vi "COD主界面（列队使用）.vi"() -> (8 "多列列表框":i32(listbox))   [LabVIEW 2016, in "斯坦道CODMn.lvlib"]
uses:
  <vilib>/Analysis/6fits.llb/Curve Fitting Criteria.ctl
  <vilib>/Utility/miscctls.llb/LVPointTypeDef.ctl
  <vilib>/Utility/config.llb/Read Key (I32).vi
  <vilib>/Utility/config.llb/Read Key (Double).vi
  <vilib>/Utility/config.llb/Read Key (Boolean).vi
  <vilib>/Utility/config.llb/Write Key (Double).vi
  <vilib>/Utility/config.llb/Write Key (Boolean).vi
  <vilib>/Utility/config.llb/Write Key (I32).vi
  <vilib>/Waveform/WDTFileIO.llb/Read Waveform from File.vi
  <vilib>/ptbypt/NI_PtbyPt.lvlib
  <vilib>/Utility/config.llb/NI_LVConfig.lvlib
  <vilib>/Analysis/NI_AALPro.lvlib
panel:
  in  "远程校准量程":enum16{"L", "H"}(ring)
  in  "远程自动校准浓度":dbl
  in  "仪器参数":bool
  out "CODMn序列号":string
  out "CODMn软件版本：":string
  in  "标样核查量程选择":enum32{"H", "L", "AUTO"}(ring)=enum."AUTO"
  in  "标样浓度":dbl
  in  "零点核查量程选择":enum32{"H", "L", "AUTO"}(ring)=enum."AUTO"
  in  "零点核查浓度":dbl
  out "序列号":string
  in  "采水泵排液时间/s:":i32
  in  "采水泵润洗时间/s:":i32
  in  "采水泵沉淀时间/s:":i32
  in  "采水泵进样时间/s:":i32
  in  "常规版/认证版":enum16{"常规版", "认证版", "浮台版"}(ring)
  in  "释放串口":bool
  in  "打开串口":bool
  in  "保存参数":dbl[](array[numeric])
  out "报警数字":i16
  out "CODMn工作状态":T1(ring)
  out "ORP-K":string
  out "ORP-B":string
  out "ORP-A":string
  out "x = y?":bool
  out "稀释倍数解释":string
  in  "跨度量程选择":enum32{"H", "L", "AUTO"}(ring)=enum."AUTO"
  in  "跨度液浓度":dbl
  in  "水样":dbl
  in  "蒸馏水":dbl
  in  "标液":dbl
  in  "质控样":dbl
  in  "加标回收":dbl
  in  "草酸钠":dbl
  in  "高锰酸钾":dbl
  in  "硫酸":dbl
  out "量程解释说明":string
  in  "高切低阈值:":dbl
  in  "低切高阈值:":dbl
  in  "自动切换量程:":enum16{"关闭", "自动切换测一次", "自动切换测两次"}(ring)
  in  "修正系数":dbl
  in  "标准液浓度":dbl
  in  "温度":dbl
  in  "恒温时间":dbl
  in  "基本量程":enum16{"L", "H"}(ring)
  in  "CODMn零点核查选择":enum16{"零点核查走纯水管", "零点核查走零漂管"}(ring)
  in  "锁定按钮":bool
  in  "低量程稀释倍数:":i8=1
  in  "高量程稀释倍数:":i8=2
  in  "一键写入":bool
  in  "测量模式(公式)":u16(ring)=1 items=["水样测试"=1, "标样核查"=2, "零点核查"=3, "跨度核查"=4, "空白测试"=5, "平行样"=6, "加标回收"=7]
  out "基本量程(显示)":string
  out "测量模式(显示)":string
  out "数据时间":string
  out "断电排液标记":bool
  out "COM":string
  in  "启用5":bool
  in  "校准5":bool
  in  "泵滴定数5":dbl
  in  "浓度5":dbl
  in  "启用4":bool
  in  "校准4":bool
  in  "泵滴定数4":dbl
  in  "浓度4":dbl
  out "波形时间":timestamp
  in  "历史波形":bool
  out "滴定数-ORP值":u16[](array[numeric]) caption="数组"
  in  "关闭 3":bool
  in  "滴定曲线":bool
  out "ORP滴定曲线":u16[](graph)
  out "空白测试标记":bool
  out "跨度核查标记":bool
  out "启动选择 2":u16(ring) items=["水样测试", "标样核查", "零点核查", "跨度核查", "空白测试", "加标回收", "平行样", "校零", "校标"]
  in  "量程选择":enum16{"低量程", "高量程", "0-2量程"}(ring)
  in  "手动控制":bool
  in  "选用水样":enum16{"葡萄糖", "草酸钠"}(ring)
  in  "方程系数":cluster{"K":dbl, "b":dbl, "X^2":dbl} {"X^2" format="%#.6g"; "b" format="%#.6g"; "K" format="%#.6g"}
  out "多项式系数":dbl[](array[numeric])
  out "XY图":cluster{"X Values":dbl[], "Y Values":dbl[]}[](graph)
  in  "模型":enum32{"线性", "多项式"}(ring)
  out "启动时间":timestamp format="%<%Y/%m/%d %H:%M:%S>T"
  in  "关闭 2":bool
  out "r^2":dbl format="%.8g"
  out "拟合公式":string
  out "b":dbl format="%#.4g"
  out "K":dbl format="%#.4f"
  out "当前校准":i32
  in  "启用3":bool
  in  "启用2":bool
  in  "启用1":bool
  in  "校准3":bool
  in  "校准2":bool
  in  "校准1":bool
  in  "泵滴定数3":dbl
  in  "泵滴定数2":dbl
  in  "泵滴定数1":dbl
  in  "浓度3":dbl
  in  "浓度2":dbl
  in  "浓度1":dbl
  in  "写入":bool
  out "零点核查标记":bool
  out "排液故障":bool
  out "进水样超量程":bool
  out "标样核查标记":bool
  out "平行样测量":bool
  out "加标回收测量":bool
  out "质控样测量":bool
  out "待机":bool
  out "校标错误":bool
  out "校零错误":bool
  out "测量错误":bool
  out "草酸钠报警":bool
  out "高锰酸钾报警":bool
  out "加热故障":bool
  out "温控器故障":bool
  out "ORP故障":bool
  out "排液标记":bool
  out "故障标记":bool
  out "校标标记":bool
  out "校零标记":bool
  out "通讯状态":bool
  out "水样测量":bool
  in  "读取":bool
  in  "返回":bool
  in  "校准配置":bool
  in  "零点泵计量数 2":dbl
  in  "标度泵计量数 2":dbl
  out "标度滴定值":dbl
  out "零点滴定值":dbl
  in  "保存":bool
  in  "关闭":bool
  out "仪器时间":timestamp format="%<%Y/%m/%d %H:%M:%S>T"
  out "秒":u16
  out "分":u16
  out "COD浓度（mg/L)":dbl format="%.2g"
  out "进样管":dbl
  out "高锰酸钾":dbl
  out "草酸钠":dbl
  out "硫酸":dbl
  out "ORP显示":dbl
  out "温度":dbl
  out "加热":bool
  out "搅拌":bool
  out "进硫酸":bool
  out "进加标回收样":bool
  out "进零点核查样":bool
  out "进标液":bool
  out "进蒸馏水":bool
  out "进水样":bool
  out "进草酸钠":bool
  out "进高锰酸钾":bool
  out "定时启动":bool
  in  "启动":bool
  in  "故障清除":bool
  in  "参数配置":bool
  in  "停止":bool
  in  "单步启动":bool
  out "系统时间":timestamp
  in  "时间校准":bool
  out "模式（受控）":u16
  # "测量时间："
  # "(水样~加标回收)"
  # "mV"
  # "℃"
  # "注：遇到加热故障和排液故障时仪器不能正常启动，\n必须排查故障并点击报警清除按钮方可运行。"
  # "mg/L"
  # "基本参数设置"
  # "校零校标结果"
  # "泵计量参数设置"
  # "校零结果："
  # "校零滴定值："
  # "加热恒温温度(℃):"
  # "水样："
  # "高锰酸钾："
  # "校标结果："
  # "标度滴定值："
  # "恒温时间(分钟):"
  # "草酸钠："
  # "蒸馏水："
  # "零点泵计量值："
  # "标准液浓度(mg/L):"
  # "硫酸："
  # "标液："
  # "标度泵计量值："
  # "修正系数："
  # "跨度核查浓度："
  # "零点核查样:"
  # "基本量程(L、H)可选:"
  # "跨度量程选择："
  # "加标回收样："
  # "零点核查浓度："
  # "标样浓度："
  # "零点量程选择："
  # "标样量程选择："
  # "远程校准配置区"
  # "公式读取写入区"
  # "mg/L"
  # "是否启用"
  # "泵滴定数"
  # "浓度"
  # "辅\n助\n计\n算\n区"
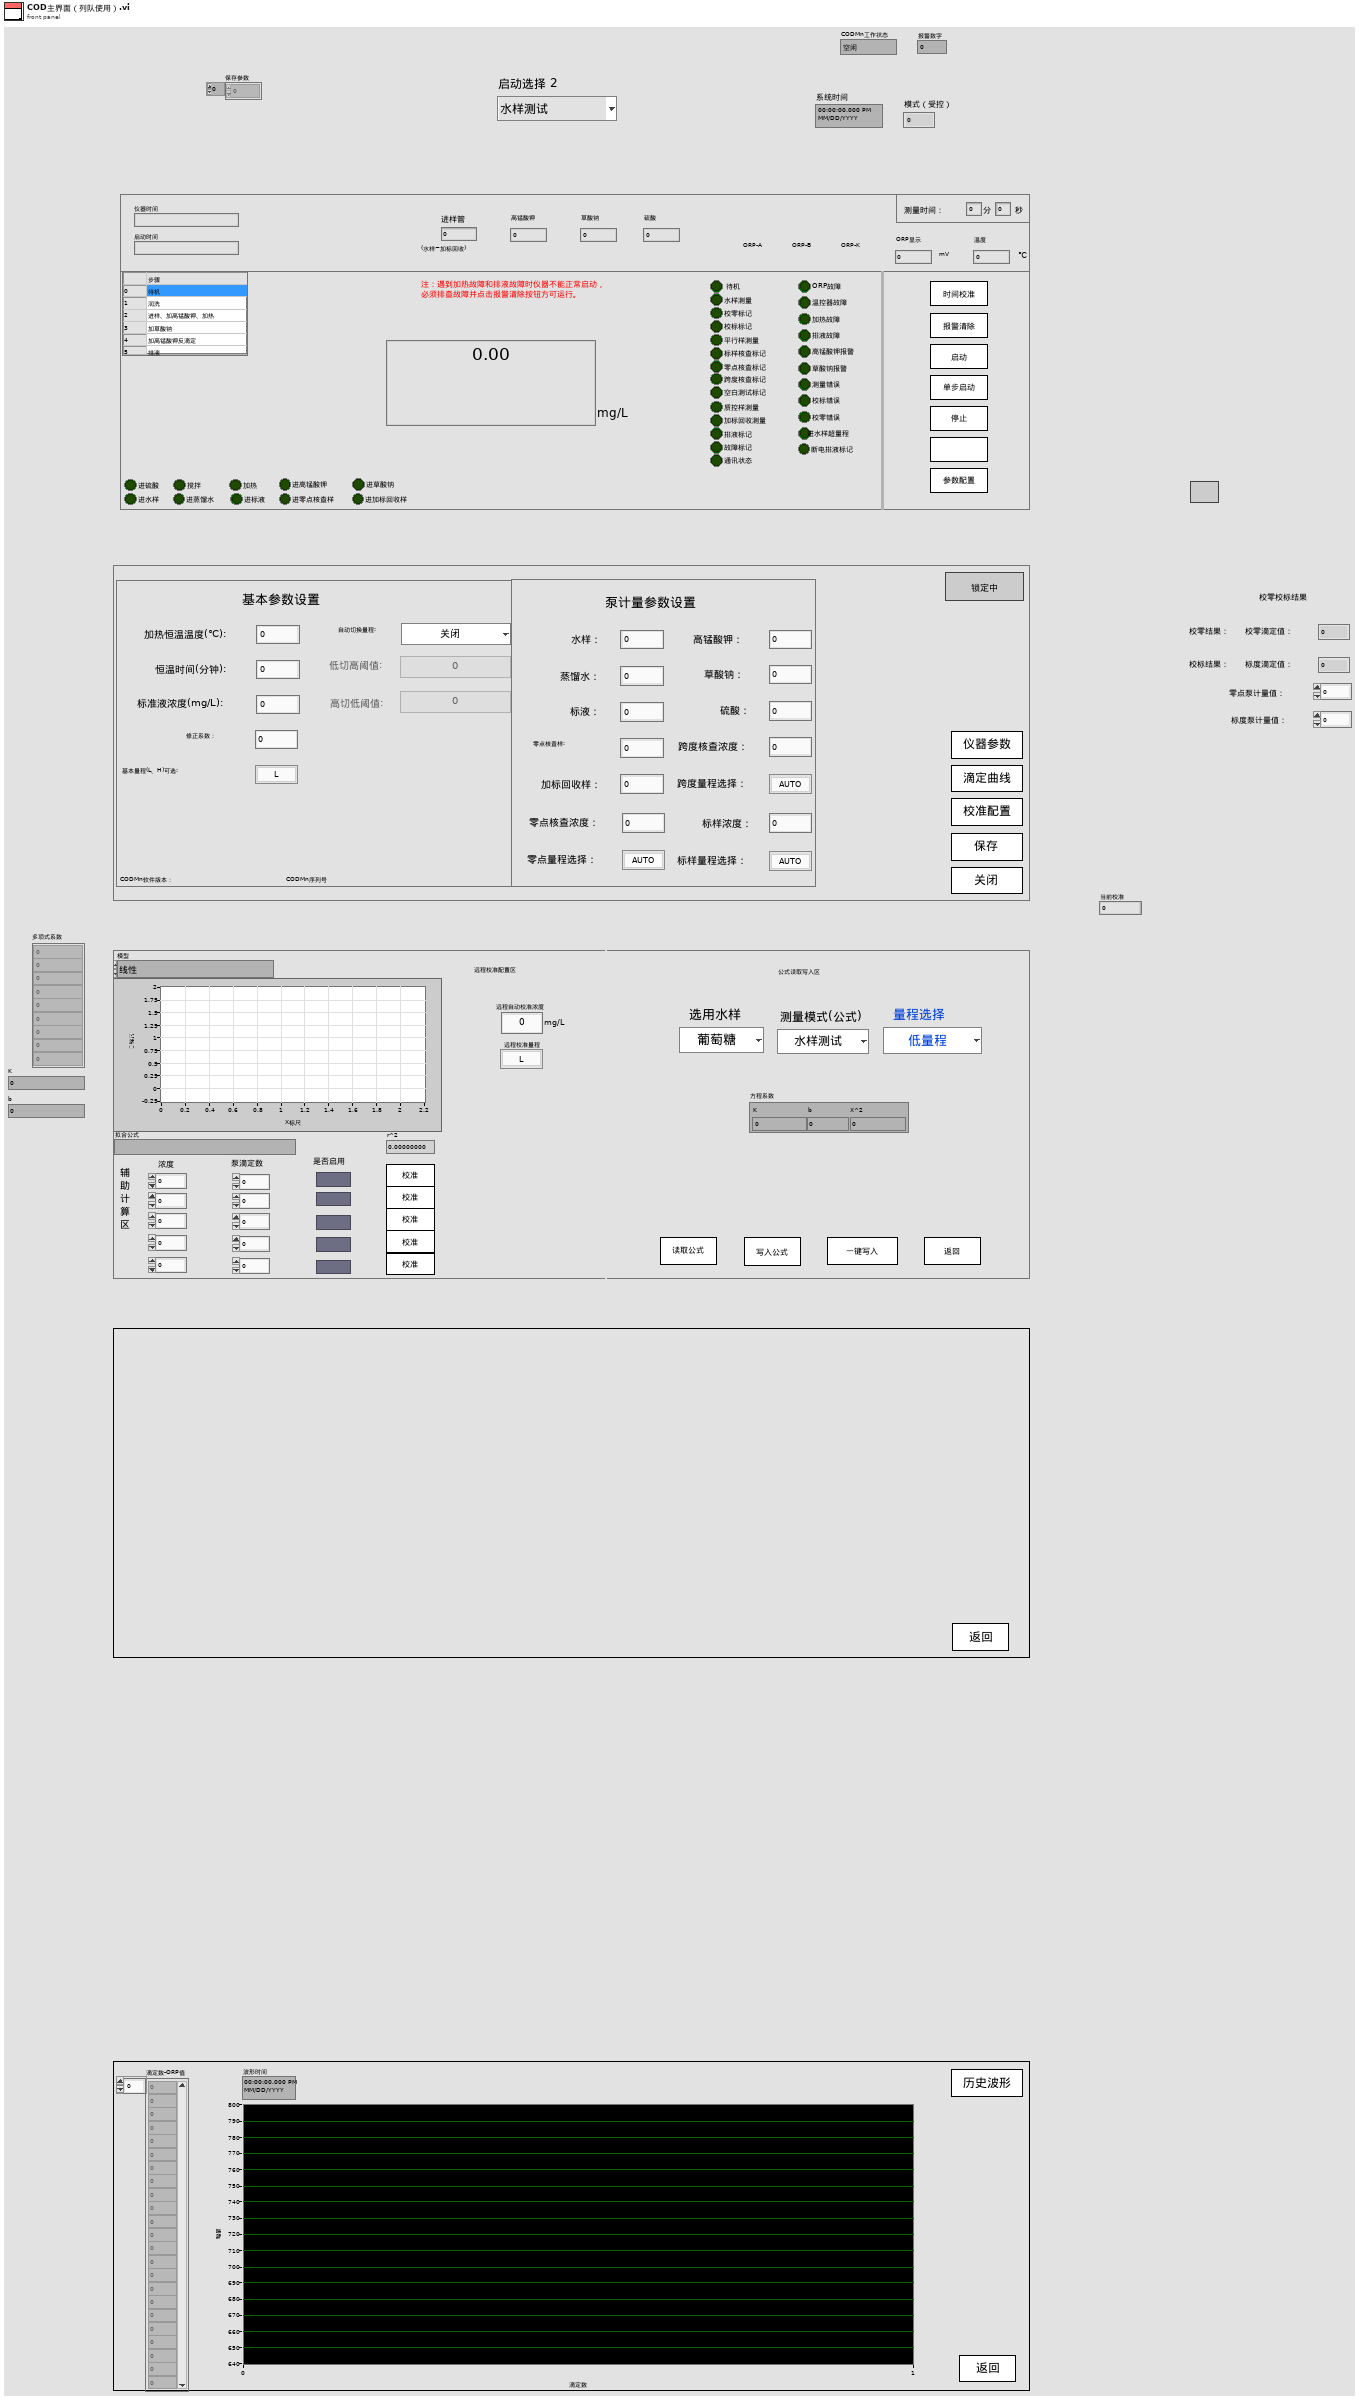
[diagram p1: front panel]
types:
  T1 = enum16{"空闲", "水样测试", "标样核查", "零点核查", "跨度核查", "空白测试", "平行样测试", "质控样", "空白校准", "标样校准", "加标回收"}
  T2 = typedef "LVPointTypeDef.ctl" = cluster{"Horizontal":i16, "Vertical":i16}
  T3 = typedef "NI_LVConfig.lvlib/Config Data RefNum.ctl" = refnum<k1>
  T4 = enum8{"Enabled", "Disabled", "Disabled and Grayed Out"}
  T5 = cluster{"仪器测试类型":enum16{"水样测试", "零点核查", "标样核查", "空白测试", "跨度核查", "加标回收", "平行样", "校零", "校标"}, "周期设置类型":enum16{"定点启动", "间隔启动"}, "定时功能启用":bool, "定时间隔":dbl, "24H周期设置":bool[]}
  T6 = typedef "NI_AALPro.lvlib/Curve Fitting Criteria.ctl" = u16
  T7 = cluster{"测量量程":dbl, "测量精度":dbl, "测量间隔":dbl, "消解温度":dbl, "消解时长":dbl, "空白校准时间":timestamp, "曲线截距":dbl, "曲线斜率":dbl, "测量检出限":dbl, "测量信号值":dbl, "线性相关系数":dbl, "二次多项式系数":dbl, "标样校准时间":timestamp, "单位":u16}
  T8 = cluster{"时间":timestamp, "测量模式":string, "数据类型":string, "检测值":sgl, "单位":string, "数据标识":string, "因子编码":string, "标样参考值":sgl, "ORP-A":sgl, "ORP-B":sgl, "ORP-K":sgl, "COD滴定值":sgl, "高锰酸钾滴定数":sgl, "温度":sgl, "量程":sgl, "LastTime":timestamp}
  T9 = cluster{"因子编码":u32, "单位":u16, "标样参考值":sgl, "水样数据时间":timestamp, "水样实测值":sgl, "水样数据标识":string, "标样数据时间":timestamp, "标样实测值":sgl, "标样数据标识":string, "空白数据时间":timestamp, "空白实测值":sgl, "空白数据标识":string, "零点核查数据时间":timestamp, "零点核查实测值":sgl, "零点核查数据标识":string, "跨度核查数据时间":timestamp, "跨度核查实测值":sgl, "跨度核查数据标识":string, "加标回收数据时间":timestamp, "加标回收实测值":sgl, "加标回收数据标识":string, "平行样数据时间":timestamp, "平行样实测值":sgl, "平行样数据标识":string}
  T10 = cluster{"数组 2[0]":sgl, "数组 2[1]":sgl, "数组 2[2]":sgl, "数组 2[3]":sgl, "数组 2[4]":sgl, "数组 2[5]":sgl, "数组 2[6]":sgl, "数组 2[7]":sgl, "数组 2[8]":sgl, "数组 2[9]":sgl, "数组 2[10]":sgl, "数组 2[11]":sgl, "数组 2[12]":sgl, "数组 2[13]":sgl, "数组 2[14]":sgl, "数组 2[15]":sgl, "数组 2[16]":sgl, "数组 2[17]":sgl, "数组 2[18]":sgl, "数组 2[19]":sgl, "数组 2[20]":sgl, "数组 2[21]":sgl, "数组 2[22]":sgl, "数组 2[23]":sgl, "数组 2[24]":sgl, "数组 2[25]":sgl, "数组 2[26]":sgl, "数组 2[27]":sgl, "数组 2[28]":sgl, "数组 2[29]":sgl, "数组 2[30]":sgl, "数组 2[31]":sgl, "数组 2[32]":sgl, "数组 2[33]":sgl, "数组 2[34]":sgl, "数组 2[35]":sgl, "数组 2[36]":sgl, "数组 2[37]":sgl, "数组 2[38]":sgl, "数组 2[39]":sgl, "数组 2[40]":sgl, "数组 2[41]":sgl}
  T11 = cluster{"ORP故障":bool, "温控器故障":bool, "加热故障":bool, "高锰酸钾报警":bool, "草酸钠报警":bool, "测量错误":bool, "校零错误":bool, "校标错误":bool, " 进水样超量程":bool, "排液阀故障":bool}
  T12 = cluster{"时间标识":timestamp, "参数":string, "日志信息":string, "流程参数":string}
  T13 = cluster{"确定":bool, "测量量程":dbl, "测量精度":dbl, "测量间隔":dbl, "消解温度":dbl, "消解时长":dbl, "空白校准时间":timestamp, "曲线截距":dbl, "曲线斜率":dbl, "测量检出限":dbl, "测量信号值":dbl, "线性相关系数":dbl, "二次多项式系数":dbl, "标样校准时间":timestamp, "单位":u16}
  T14 = cluster{"时间标识":timestamp, "设备":string, "日志信息":string, "流程参数":string}
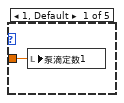
[diagram p4: hidden frame]
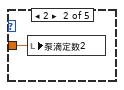
[diagram p5: hidden frame]
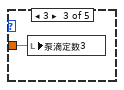
[diagram p6: hidden frame]
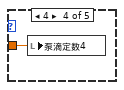
[diagram p7: hidden frame]
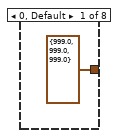
[diagram p12: hidden frame]
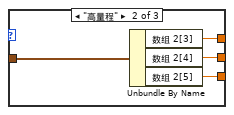
[diagram p13: hidden frame]
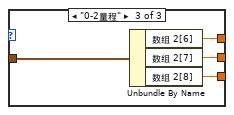
[diagram p14: hidden frame]
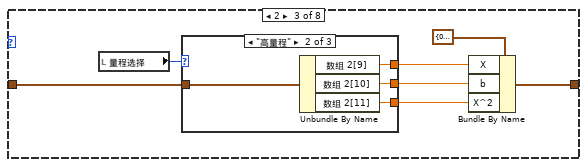
[diagram p15: hidden frame]
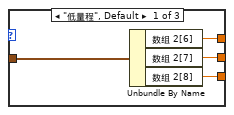
[diagram p16: hidden frame]
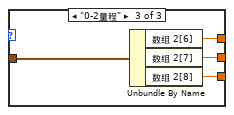
[diagram p17: hidden frame]
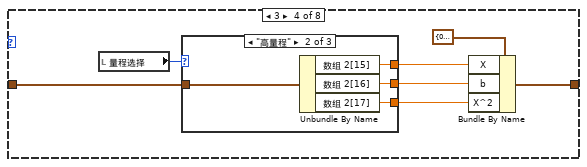
[diagram p18: hidden frame]
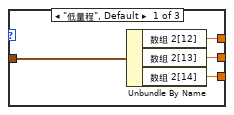
[diagram p19: hidden frame]
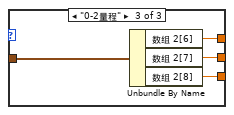
[diagram p20: hidden frame]
diagram:
  n1 = flat-sequence {
    tunnel: [w57] -> w39
    tunnel: [errorcluster {"status"=FALSE, "code"=0, "source"=""} ("错误输出")] -> w37
    frame #0 {
      n2 = global read "COD内部交互全局.vi" "序列号:"() -> (w54:string)
      "序列号" <- w54
      n3 = global write "COD内部交互全局.vi" "量程切换次数"(u8 0 ("量程切换次数")) -> ()
      n4 = global write "COD内部交互全局.vi" "切换量程连续测两次"(FALSE ("切换量程连续测两次")) -> ()
      n5 = property on="窗格" class="Pane"("Origin"=T2 {"Horizontal"=0, "Vertical"=0} ("原点")) -> ()  [unwired: 2 in, 2 out]
      n6 = local write "量程选择"(enum16{"低量程", "高量程", "0-2量程"}."低量程" ("量程选择")) -> ()
      n7 = local write "选用水样"(enum16{"葡萄糖", "草酸钠"}."葡萄糖" ("选用水样")) -> ()
      n8 = Empty String/Path?(string/path=w54) -> (empty?=w56:bool)
      n9 = case shown="真" w56 {
        tunnel: w54 -> [w72 _]
        tunnel: [w71 "data\\Set.ini" ("名称或相对路径")] -> w55
        frame False {
          # "与生产用上位机交互"
          n10 = Concatenate Strings("data\\" ("字符串"), "序列号" ("字符串"), w72, "Set.ini" ("名称或相对路径")) -> (w71:string)
        }
        frame True {
        }
      }
      n11 = call <vilib>:"Application Directory.vi"() -> ("Application Directory"=w66:path)
      n12 = global write "COD内部交互全局.vi" "配置文件ini"(w55) -> ()
      n13 = Build Path(base path=w66, name or relative path=w55) -> (appended path=w65:path)
      n14 = call <vilib>:"Open Config Data.vi"("configuration file path"=w65) -> ("error out"=w61:errorcluster, "refnum"=w64:T3)  [unwired: 8 in, 1 out]
      n15 = vi-ref "斯坦道CODMn.lvlib:CODMn断电保存全局变量.vi"() -> (w63:refnum<vi>)
      n16 = call <userlib>:"Read Panel from INI__ogtk.vi"("error in (no error)"=w61, "VI ref"=w63, "refnum"=w64) -> ("error out"=w60:errorcluster, "refnum out"=w62:T3)  [unwired: 7 in]
      n17 = call <vilib>:"Close Config Data.vi"("error in (no error)"=w60, "refnum"=w62) -> ("error out"=w59:errorcluster, "file path"=w58:path)  [unwired: 8 in]
      n18 = Open/Create/Replace File(file path (use dialog)=w58, error in=w59) -> (error out=w57:errorcluster)  [unwired: 4 in, 2 out]
      "稀释倍数解释" <- "稀释倍数解释：\n稀释倍数选择1，表示不稀释\n默认低量程系数倍数1，高量程系数倍数2\n则低量程为0~8，高量程为0~16" ("稀释倍数解释")
    }
  }
  n19 = while {
    stop <- FALSE stop-if-true
    # "数字键盘输入"
    n20 = event shown="[25] \"泵滴定数3\": 鼠标按下" {
      selector: _ -> [_ _ _ _ _ _ _ _ _ _ _ _ _ _ _ _ _ _ _ _ _ _ _ _ _ _ _ _ _ _]
      dyn-events: _ -> [_ _ _ _ _ _ _ _ _ _ _ _ _ _ _ _ _ _ _ _ _ _ _ _ _ _ _ _ _ _]
      timeout: _ -> [_ _ _ _ _ _ _ _ _ _ _ _ _ _ _ _ _ _ _ _ _ _ _ _ _ _ _ _ _ _]
      event Timeout {
        n21 = event-data() -> ()  [unwired: 1 in, 3 out]
      }
      event "温度": Mouse Down {
        n22 = event-data() -> ()  [unwired: 1 in, 8 out]
        n23 = local read "温度"() -> (w79:dbl)
        n24 = call "数字键盘.vi"("OldNumber"=w79) -> ("NewNumber"=w78:sgl)
        n25 = local write "温度"(w78) -> ()
      }
      event "恒温时间": Mouse Down {
        n26 = event-data() -> ()  [unwired: 1 in, 8 out]
        n27 = local read "恒温时间"() -> (w80:dbl)
        n28 = call "数字键盘.vi"("OldNumber"=w80) -> ("NewNumber"=w81:sgl)
        n29 = local write "恒温时间"(w81) -> ()
      }
      event "标准液浓度": Mouse Down {
        n30 = event-data() -> ()  [unwired: 1 in, 8 out]
        n31 = local read "标准液浓度"() -> (w83:dbl)
        n32 = call "数字键盘.vi"("OldNumber"=w83) -> ("NewNumber"=w82:sgl)
        n33 = local write "标准液浓度"(w82) -> ()
      }
      event "修正系数": Mouse Down {
        n34 = event-data() -> ()  [unwired: 1 in, 8 out]
        n35 = local read "修正系数"() -> (w84:dbl)
        n36 = call "数字键盘.vi"("OldNumber"=w84) -> ("NewNumber"=w85:sgl)
        n37 = local write "修正系数"(w85) -> ()
      }
      event "水样": Mouse Down {
        n38 = event-data() -> ()  [unwired: 1 in, 8 out]
        n39 = local read "水样"() -> (w86:dbl)
        n40 = call "数字键盘.vi"("OldNumber"=w86) -> ("NewNumber"=w87:sgl)
        n41 = local write "水样"(w87) -> ()
      }
      event "蒸馏水": Mouse Down {
        n42 = event-data() -> ()  [unwired: 1 in, 8 out]
        n43 = local read "蒸馏水"() -> (w88:dbl)
        n44 = call "数字键盘.vi"("OldNumber"=w88) -> ("NewNumber"=w89:sgl)
        n45 = local write "蒸馏水"(w89) -> ()
      }
      event "标液": Mouse Down {
        n46 = event-data() -> ()  [unwired: 1 in, 8 out]
        n47 = local read "标液"() -> (w90:dbl)
        n48 = call "数字键盘.vi"("OldNumber"=w90) -> ("NewNumber"=w91:sgl)
        n49 = local write "标液"(w91) -> ()
      }
      event "质控样": Mouse Down {
        n50 = event-data() -> ()  [unwired: 1 in, 8 out]
        n51 = local read "质控样"() -> (w92:dbl)
        n52 = call "数字键盘.vi"("OldNumber"=w92) -> ("NewNumber"=w93:sgl)
        n53 = local write "质控样"(w93) -> ()
      }
      event "加标回收": Mouse Down {
        n54 = event-data() -> ()  [unwired: 1 in, 8 out]
        n55 = local read "加标回收"() -> (w94:dbl)
        n56 = call "数字键盘.vi"("OldNumber"=w94) -> ("NewNumber"=w95:sgl)
        n57 = local write "加标回收"(w95) -> ()
      }
      event "草酸钠": Mouse Down {
        n58 = event-data() -> ()  [unwired: 1 in, 8 out]
        n59 = local read "草酸钠"() -> (w96:dbl)
        n60 = call "数字键盘.vi"("OldNumber"=w96) -> ("NewNumber"=w97:sgl)
        n61 = local write "草酸钠"(w97) -> ()
      }
      event "高锰酸钾": Mouse Down {
        n62 = event-data() -> ()  [unwired: 1 in, 8 out]
        n63 = local read "高锰酸钾"() -> (w98:dbl)
        n64 = call "数字键盘.vi"("OldNumber"=w98) -> ("NewNumber"=w99:sgl)
        n65 = local write "高锰酸钾"(w99) -> ()
      }
      event "硫酸": Mouse Down {
        n66 = event-data() -> ()  [unwired: 1 in, 8 out]
        n67 = local read "硫酸"() -> (w100:dbl)
        n68 = call "数字键盘.vi"("OldNumber"=w100) -> ("NewNumber"=w101:sgl)
        n69 = local write "硫酸"(w101) -> ()
      }
      event "零点泵计量数 2": Mouse Down {
        n70 = event-data() -> ()  [unwired: 1 in, 8 out]
        n71 = local read "零点泵计量数 2"() -> (w102:dbl)
        n72 = call "数字键盘.vi"("OldNumber"=w102) -> ("NewNumber"=w103:sgl)
        n73 = local write "零点泵计量数 2"(w103) -> ()
      }
      event "标度泵计量数 2": Mouse Down {
        n74 = event-data() -> ()  [unwired: 1 in, 8 out]
        n75 = local read "标度泵计量数 2"() -> (w104:dbl)
        n76 = call "数字键盘.vi"("OldNumber"=w104) -> ("NewNumber"=w105:sgl)
        n77 = local write "标度泵计量数 2"(w105) -> ()
      }
      event "高量程稀释倍数:": Mouse Down {
        n78 = event-data() -> ()  [unwired: 1 in, 8 out]
        n79 = local read "高量程稀释倍数:"() -> (w107:i8)
        n80 = call "数字键盘.vi"("OldNumber"=w107) -> ("NewNumber"=w106:sgl)
        n81 = local write "高量程稀释倍数:"(w106) -> ()
      }
      event "低量程稀释倍数:": Mouse Down {
        n82 = event-data() -> ()  [unwired: 1 in, 8 out]
        n83 = local read "低量程稀释倍数:"() -> (w109:i8)
        n84 = call "数字键盘.vi"("OldNumber"=w109) -> ("NewNumber"=w108:sgl)
        n85 = local write "低量程稀释倍数:"(w108) -> ()
      }
      event "浓度1": Mouse Down {
        n86 = event-data() -> ()  [unwired: 1 in, 8 out]
        n87 = local read "浓度1"() -> (w111:dbl)
        n88 = call "数字键盘.vi"("OldNumber"=w111) -> ("NewNumber"=w110:sgl)
        n89 = property on="浓度1" class="DigNum (严格)"("Val(Sgnl)"=w110) -> ()  [unwired: 2 in, 2 out]
      }
      event "浓度2": Mouse Down {
        n90 = event-data() -> ()  [unwired: 1 in, 8 out]
        n91 = local read "浓度2"() -> (w113:dbl)
        n92 = call "数字键盘.vi"("OldNumber"=w113) -> ("NewNumber"=w112:sgl)
        n93 = property on="浓度2" class="DigNum (严格)"("Val(Sgnl)"=w112) -> ()  [unwired: 2 in, 2 out]
      }
      event "浓度3": Mouse Down {
        n94 = event-data() -> ()  [unwired: 1 in, 8 out]
        n95 = local read "浓度3"() -> (w115:dbl)
        n96 = call "数字键盘.vi"("OldNumber"=w115) -> ("NewNumber"=w114:sgl)
        n97 = property on="浓度3" class="DigNum (严格)"("Val(Sgnl)"=w114) -> ()  [unwired: 2 in, 2 out]
      }
      event "浓度4": Mouse Down {
        n98 = event-data() -> ()  [unwired: 1 in, 8 out]
        n99 = local read "浓度4"() -> (w117:dbl)
        n100 = call "数字键盘.vi"("OldNumber"=w117) -> ("NewNumber"=w116:sgl)
        n101 = property on="浓度4" class="DigNum (严格)"("Val(Sgnl)"=w116) -> ()  [unwired: 2 in, 2 out]
      }
      event "浓度5": Mouse Down {
        n102 = event-data() -> ()  [unwired: 1 in, 8 out]
        n103 = local read "浓度5"() -> (w119:dbl)
        n104 = call "数字键盘.vi"("OldNumber"=w119) -> ("NewNumber"=w118:sgl)
        n105 = property on="浓度5" class="DigNum (严格)"("Val(Sgnl)"=w118) -> ()  [unwired: 2 in, 2 out]
      }
      event "跨度液浓度", "零点核查浓度", "标样浓度": Mouse Down {
        n106 = event-data() -> ("CtlRef"=w123:refnum<vi>)  [unwired: 1 in, 7 out]
        n107 = property class="DigNum (严格)"(reference=w123) -> (reference out=w120:refnum<vi>, "Value"=w122:dbl)  [unwired: 1 in, 1 out]
        n108 = call "数字键盘.vi"("OldNumber"=w122) -> ("NewNumber"=w121:sgl)
        n109 = property class="DigNum (严格)"(reference=w120, "Val(Sgnl)"=w121) -> ()  [unwired: 1 in, 2 out]
      }
      event "泵滴定数1": Mouse Down {
        n110 = event-data() -> ()  [unwired: 1 in, 8 out]
        n111 = local read "泵滴定数1"() -> (w125:dbl)
        n112 = call "数字键盘.vi"("OldNumber"=w125) -> ("NewNumber"=w124:sgl)
        n113 = property on="泵滴定数1" class="DigNum (严格)"("Val(Sgnl)"=w124) -> ()  [unwired: 2 in, 2 out]
      }
      event "泵滴定数2": Mouse Down {
        n114 = event-data() -> ()  [unwired: 1 in, 8 out]
        n115 = local read "泵滴定数2"() -> (w127:dbl)
        n116 = call "数字键盘.vi"("OldNumber"=w127) -> ("NewNumber"=w126:sgl)
        n117 = property on="泵滴定数2" class="DigNum (严格)"("Val(Sgnl)"=w126) -> ()  [unwired: 2 in, 2 out]
      }
      event "泵滴定数3": Mouse Down {
        n118 = event-data() -> ()  [unwired: 1 in, 8 out]
        n119 = local read "泵滴定数3"() -> (w129:dbl)
        n120 = call "数字键盘.vi"("OldNumber"=w129) -> ("NewNumber"=w128:sgl)
        n121 = property on="泵滴定数3" class="DigNum (严格)"("Val(Sgnl)"=w128) -> ()  [unwired: 2 in, 2 out]
      }
      event "泵滴定数4": Mouse Down {
        n122 = event-data() -> ()  [unwired: 1 in, 8 out]
        n123 = local read "泵滴定数4"() -> (w131:dbl)
        n124 = call "数字键盘.vi"("OldNumber"=w131) -> ("NewNumber"=w130:sgl)
        n125 = property on="泵滴定数4" class="DigNum (严格)"("Val(Sgnl)"=w130) -> ()  [unwired: 2 in, 2 out]
      }
      event "泵滴定数5": Mouse Down {
        n126 = event-data() -> ()  [unwired: 1 in, 8 out]
        n127 = local read "泵滴定数5"() -> (w133:dbl)
        n128 = call "数字键盘.vi"("OldNumber"=w133) -> ("NewNumber"=w132:sgl)
        n129 = property on="泵滴定数5" class="DigNum (严格)"("Val(Sgnl)"=w132) -> ()  [unwired: 2 in, 2 out]
      }
      event "低切高阈值:", "高切低阈值:": Mouse Down {
        n130 = event-data() -> ("CtlRef"=w137:refnum<vi>)  [unwired: 1 in, 7 out]
        n131 = property class="DigNum (严格)"(reference=w137) -> (reference out=w136:refnum<vi>, "Value"=w135:dbl)  [unwired: 1 in, 1 out]
        n132 = call "数字键盘.vi"("OldNumber"=w135) -> ("NewNumber"=w134:sgl)
        n133 = property class="DigNum (严格)"(reference=w136, "Val(Sgnl)"=w134) -> ()  [unwired: 1 in, 2 out]
      }
      event "远程自动校准浓度": Mouse Down {
        n134 = event-data() -> ("CtlRef"=w138:refnum<vi>)  [unwired: 1 in, 7 out]
        n135 = property class="DigNum (严格)"(reference=w138) -> (reference out=w141:refnum<vi>, "Value"=w140:dbl)  [unwired: 1 in, 1 out]
        n136 = call "数字键盘.vi"("OldNumber"=w140) -> ("NewNumber"=w139:sgl)
        n137 = property class="DigNum (严格)"(reference=w141, "Val(Sgnl)"=w139) -> ()  [unwired: 1 in, 2 out]
      }
    }
  }
  n138 = while {
    stop <- FALSE stop-if-true
    # "赋值循环"
    n139 = flat-sequence {
      frame #0 {
        # "局部变量给内部交互用全局变量"
        n140 = local read "温度"() -> (w171:dbl)
        n141 = local read "多列列表框"() -> (w178:i32)
        n142 = local read "标准液浓度"() -> (w176:dbl)
        n143 = local read "ORP显示"() -> (w169:dbl)
        n144 = local read "当前校准"() -> (w170:i32)
        n145 = local read "故障标记"() -> (w179:bool)
        n146 = local read "高锰酸钾"() -> (w172:dbl)
        n147 = global write "COD内部交互全局.vi" "实时温度"(w171) -> ()
        n148 = local read "COD浓度（mg/L)"() -> (w177:dbl)
        n149 = local read "CODMn工作状态"() -> (w180:T1)
        n150 = local read "高锰酸钾报警"() -> (w174:bool)
        n151 = local read "断电排液标记"() -> (w173:bool)
        n152 = global write "COD内部交互全局.vi" "当前校准"(w170) -> ()
        n153 = global write "运行时序全局变量.vi" "多列列表框"(w178) -> ()
        n154 = global write "COD内部交互全局.vi" "故障标记"(w179) -> ()
        n155 = global write "COD内部交互全局.vi" "ORP显示"(w169) -> ()
        n156 = global write "COD浓度全局变量.vi" "标准液浓度"(w176) -> ()
        n157 = global write "COD内部交互全局.vi" "高锰酸钾"(w172) -> ()
        n158 = local read "待机"() -> (w175:bool)
        n159 = global write "COD内部交互全局.vi" "待机"(w175) -> ()
        n160 = global write "COD测量模式全局.vi" "CODMn工作状态"(w180) -> ()
        n161 = global write "COD内部交互全局.vi" "高锰酸钾报警"(w174) -> ()
        n162 = global write "COD内部交互全局.vi" "断电排液标记"(w173) -> ()
        n163 = global write "COD浓度全局变量.vi" "COD浓度（mg/L)"(w177) -> ()
      }
    }
    n164 = flat-sequence {
      frame #0 {
        # "断电保存全局给局部变量"
        n165 = global read "CODMn断电保存全局变量.vi" "高切低阈值:"() -> (w510:dbl)
        n166 = global read "CODMn断电保存全局变量.vi" "低切高阈值:"() -> (w509:dbl)
        n167 = global read "CODMn断电保存全局变量.vi" "跨度液浓度"() -> (w507:dbl)
        n168 = global read "COD内部交互全局.vi" "波形时间"() -> (w496:timestamp)
        n169 = global read "CODMn断电保存全局变量.vi" "启动时间"() -> (→"启动时间":timestamp)
        n170 = global read "CODMn断电保存全局变量.vi" "标样浓度"() -> (w505:dbl)
        n171 = global read "CODMn断电保存全局变量.vi" "定时控制"() -> (w500:T5)
        n172 = global read "CODMn断电保存全局变量.vi" "标样核查量程选择"() -> (w502:enum32{"H", "L", "AUTO"})
        n173 = global read "CODMn断电保存全局变量.vi" "零点核查量程选择"() -> (w504:enum32{"H", "L", "AUTO"})
        n174 = global read "CODMn断电保存全局变量.vi" "测量模式(公式)"() -> (w512:u16)
        n175 = global read "COD内部交互全局.vi" "滴定数-ORP值"() -> (→"滴定数-ORP值":u16[])
        n176 = global read "CODMn断电保存全局变量.vi" "常规版/认证版"() -> (w506:enum16{"常规版", "认证版", "浮台版"})
        n177 = global read "CODMn断电保存全局变量.vi" "自动切换量程:"() -> (w508:enum16{"关闭", "自动切换测一次", "自动切换测两次"})
        n178 = global read "CODMn断电保存全局变量.vi" "零点核查浓度"() -> (w503:dbl)
        n179 = global read "COD内部交互全局.vi" "ORP滴定曲线"() -> (→"ORP滴定曲线":u16[])
        n180 = local write "高切低阈值:"(w510) -> ()
        n181 = local write "波形时间"(w496) -> ()
        n182 = local write "标样浓度"(w505) -> ()
        n183 = Unbundle By Name(w500) -> ("定时功能启用"=→"定时启动":bool)
        n184 = local write "跨度液浓度"(w507) -> ()
        n185 = local write "低切高阈值:"(w509) -> ()
        n186 = global read "CODMn断电保存全局变量.vi" "CODMn跨度量程选择"() -> (w511:enum32{"H", "L", "AUTO"})
        n187 = local write "标样核查量程选择"(w502) -> ()
        n188 = local write "自动切换量程:"(w508) -> ()
        n189 = local write "常规版/认证版"(w506) -> ()
        n190 = local write "零点核查浓度"(w503) -> ()
        n191 = local write "零点核查量程选择"(w504) -> ()
        n192 = local write "测量模式(公式)"(w512) -> ()
        n193 = local write "跨度量程选择"(w511) -> ()
      }
    }
    n194 = flat-sequence {
      frame #0 {
        # "保存参数赋值"
        n195 = Multiply(x="温度", y=10.0) -> (x*y=w154:dbl)
        n196 = Multiply(x="标准液浓度", y=100.0) -> (x*y=w148:dbl)
        n197 = Multiply(x="修正系数", y=100.0) -> (x*y=w151:dbl)
        n198 = Build Array(w154, "恒温时间", w148, w151, "基本量程", "水样", "蒸馏水", "标液", "质控样", "加标回收", "高锰酸钾", "草酸钠", "硫酸", "零点泵计量数 2", "标度泵计量数 2", "高量程稀释倍数:", "低量程稀释倍数:", "CODMn零点核查选择") -> (w145:dbl[])
        n199 = local write "保存参数"(w145) -> ()
      }
    }
    n200 = flat-sequence {
      frame #0 {
        # "显示量程说明"
        n201 = global read "COD内部交互全局.vi" "通讯状态"() -> (→"通讯状态":bool)
        n202 = global read "CODMn断电保存全局变量.vi" "MB通信方式选择"() -> (w513:enum16{"串口", "TCP"})
        n203 = local read "低量程稀释倍数:"() -> (w527:i8)
        n204 = local read "高量程稀释倍数:"() -> (w517:i8)
        n205 = case shown="\"TCP\"" w513 {
          tunnel: [w530 w531] -> w518
          frame "串口", Default {
            n206 = global read "CODMn断电保存全局变量.vi" "VISA resource name"() -> (w530:refnum<visa-resource-name>)
          }
          frame "TCP" {
            n207 = global read "CODMn断电保存全局变量.vi" "IP"() -> (w531:string)
          }
        }
        "COM" <- w518
        n208 = Multiply(x=w527, y=i8 8) -> (x*y=w519:i8)
        n209 = Multiply(x=w517, y=i8 8) -> (x*y=w515:i8)
        n210 = Number To Decimal String(number=w519) -> (decimal integer string=w524:string)  [unwired: 1 in]
        n211 = Number To Decimal String(number=w515) -> (decimal integer string=w522:string)  [unwired: 1 in]
        n212 = Concatenate Strings("L低量程范围:0~" ("量程解释说明"), w524, "(mg/L)\n\nH高量程范围:" ("量程解释说明"), "0" ("字符串"), "~" ("量程解释说明"), w522, "(mg/L)" ("量程解释说明")) -> (→"量程解释说明":string)
      }
    }
    n213 = flat-sequence {
      frame #0 {
        # "参数赋值（只在读取参数时候改变一次）"
        n214 = global read "COD内部交互全局.vi" "读取浮台参数显示"() -> (w182:bool)
        n215 = global read "COD内部交互全局.vi" "读取浮台参数"() -> (w181:u16[])
        n216 = global read "COD内部交互全局.vi" "读取参数显示"() -> (w183:bool)
        n217 = global read "COD内部交互全局.vi" "读取参数"() -> (w184:u16[])
        n218 = case shown="真" w182 {
          tunnel: w181 -> [_ w190]
          frame False {
          }
          frame True {
            n219 = Index Array(array=w190) -> (element #1=w189:u16, element #2=w188:u16, element #3=w187:u16, element #4=w186:u16)  [unwired: 4 in]
            n220 = global write "COD内部交互全局.vi" "读取浮台参数显示"(FALSE ("读取参数显示")) -> ()
            n221 = local write "采水泵进样时间/s:"(w189) -> ()
            n222 = local write "采水泵润洗时间/s:"(w188) -> ()
            n223 = local write "采水泵沉淀时间/s:"(w187) -> ()
            n224 = local write "采水泵排液时间/s:"(w186) -> ()
          }
        }
        n225 = case shown="真" w183 {
          tunnel: w184 -> [_ w207]
          frame False {
          }
          frame True {
            n226 = Index Array(array=w207) -> (element #1=w219:u16, element #2=w231:u16, element #3=w212:u16, element #4=w217:u16, element #5=w215:u16, element #6=w214:u16, element #7=w230:u16, element #8=w229:u16, element #9=w228:u16, element #10=w227:u16, element #11=w226:u16, element #12=w225:u16, element #13=w224:u16, element #14=w223:u16, element #15=w222:u16, element #16=w210:u16, element #17=w209:u16, element #18=w208:u16, element #19=w205:u16, element #20=w204:u16, element #21=w203:u16, element #22=w202:u16, element #23=w201:u16, element #27=w197:u16, element #28=w196:u16, element #29=w195:u16, element #30=w194:u16, element #31=w193:u16)  [unwired: 31 in, 3 out]
            n227 = global write "COD内部交互全局.vi" "读取参数显示"(FALSE ("读取参数显示")) -> ()
            n228 = local write "水样"(w214) -> ()
            n229 = local write "标液"(w229) -> ()
            n230 = local write "硫酸"(w224) -> ()
            n231 = local write "恒温时间"(w231) -> ()
            n232 = local write "基本量程"(w215) -> ()
            n233 = local write "蒸馏水"(w230) -> ()
            n234 = local write "质控样"(w228) -> ()
            n235 = local write "加标回收"(w227) -> ()
            n236 = local write "高锰酸钾"(w226) -> ()
            n237 = local write "草酸钠"(w225) -> ()
            n238 = local write "零点泵计量数 2"(w223) -> ()
            n239 = local write "标度泵计量数 2"(w222) -> ()
            n240 = local write "高量程稀释倍数:"(w210) -> ()
            n241 = local write "低量程稀释倍数:"(w209) -> ()
            n242 = local write "CODMn零点核查选择"(w208) -> ()
            n243 = Build Array(w205, w204, w203, w202, w201) -> (w200:u16[])
            n244 = Build Array(w197, w196, w195, w194, w193) -> (w192:u16[])
            n245 = Divide(x=w219, y=u16 10) -> (x/y=w220:dbl)
            n246 = Divide(x=w212, y=u16 100) -> (x/y=w211:dbl)
            n247 = Divide(x=w217, y=u16 100) -> (x/y=w216:dbl)
            n248 = local write "温度"(w220) -> ()
            n249 = local write "标准液浓度"(w211) -> ()
            n250 = local write "修正系数"(w216) -> ()
            n251 = call "HexToString.vi"("数组"=w192) -> ("字符串"=→"CODMn序列号":string)  [unwired: 10 in]
            n252 = call "FATEK_HexToString.vi"("数组"=w200) -> ("STRING"=w199:string[])  [unwired: 10 in]
            n253 = Index Array(array=w199) -> (element=→"CODMn软件版本：":string)  [unwired: 1 in]
          }
        }
      }
    }
    n254 = flat-sequence {
      frame #0 {
        # "权限隐藏和显示功能"
        n255 = local read "x = y?"() -> (w532:bool)
        n256 = property on="释放串口" class="Bool"("Visible"=w532) -> ()  [unwired: 2 in, 2 out]
        n257 = property on="打开串口" class="Bool"("Visible"=w532) -> ()  [unwired: 2 in, 2 out]
        n258 = local read "常规版/认证版"() -> (w537:enum16{"常规版", "认证版", "浮台版"})
        n259 = property on="常规版/认证版" class="Enum (严格)"("Visible"=w532) -> ()  [unwired: 2 in, 2 out]
        n260 = property on="CODMn零点核查选择" class="Enum (严格)"("Visible"=w532) -> ()  [unwired: 2 in, 2 out]
        n261 = property on="低量程稀释倍数:" class="DigNum (严格)"("Visible"=w532) -> ()  [unwired: 2 in, 2 out]
        n262 = property on="稀释倍数解释" class="Str"("Visible"=w532) -> ()  [unwired: 2 in, 2 out]
        n263 = property on="高量程稀释倍数:" class="DigNum (严格)"("Visible"=w532) -> ()  [unwired: 2 in, 2 out]
        n264 = case shown="\"浮台版\"" w537 {
          tunnel: [T4."Enabled" ("禁用") T4."Disabled and Grayed Out" ("禁用") T4."Enabled" ("禁用")] -> w536
          tunnel: [i32[] [2] ("禁用项[]") i32[] [] ("禁用项[]") i32[] [2] ("禁用项[]")] -> w535
          tunnel: [T4."Enabled" ("禁用") T4."Disabled and Grayed Out" ("禁用") T4."Enabled" ("禁用")] -> w534
          tunnel: [FALSE FALSE TRUE] -> w533
          frame "常规版", Default {
          }
          frame "认证版" {
            w548 = u16 1 items=["水样测试"=1, "标样核查"=2, "零点核查"=3, "跨度核查"=4, "空白测试"=5, "平行样"=6, "加标回收"=7] ("测量模式(公式)")
            n265 = global write "CODMn断电保存全局变量.vi" "测量模式(公式)"(w548) -> ()
          }
          frame "浮台版" {
          }
        }
        n266 = local read "自动切换量程:"() -> (w539:enum16{"关闭", "自动切换测一次", "自动切换测两次"})
        n267 = Not Equal To 0?(x=w539) -> (x != 0?=w538:bool)
        n268 = Select(t=T4."Enabled" ("禁用"), s=w538, f=T4."Disabled and Grayed Out" ("禁用")) -> (s? t:f=w540:T4)
        n269 = property on="低切高阈值:" class="DigNum (严格)"("DisabledEnum"=w540) -> ()  [unwired: 2 in, 2 out]
        n270 = property on="高切低阈值:" class="DigNum (严格)"("DisabledEnum"=w540) -> ()  [unwired: 2 in, 2 out]
        n271 = property on="采水泵润洗时间/s:" class="DigNum (严格)"("Visible"=w533) -> ()  [unwired: 2 in, 2 out]
        n272 = property on="采水泵沉淀时间/s:" class="DigNum (严格)"("Visible"=w533) -> ()  [unwired: 2 in, 2 out]
        n273 = property on="采水泵排液时间/s:" class="DigNum (严格)"("Visible"=w533) -> ()  [unwired: 2 in, 2 out]
        n274 = property on="采水泵进样时间/s:" class="DigNum (严格)"("Visible"=w533) -> ()  [unwired: 2 in, 2 out]
        n275 = property on="一键写入" class="Bool (严格)"("DisabledEnum"=w534) -> ()  [unwired: 2 in, 2 out]
        n276 = property on="量程选择" class="Enum (严格)"("Disabled Items []"=w535) -> ()  [unwired: 2 in, 2 out]
        n277 = property on="测量模式(公式)" class="Ring (严格)"("DisabledEnum"=w536) -> ()  [unwired: 2 in, 2 out]
      }
    }
    n278 = flat-sequence {
      frame #0 {
        w404 = T6 0 items=["最小二乘", "最小绝对残差", "Bisquare"] ("method")
        # "计算线性、多项式公式"
        n279 = local read "浓度1"() -> (w407:dbl)
        n280 = local read "浓度2"() -> (w408:dbl)
        n281 = local read "浓度3"() -> (w409:dbl)
        n282 = local read "浓度4"() -> (w399:dbl)
        n283 = local read "浓度5"() -> (w398:dbl)
        n284 = Unbundle By Name("方程系数") -> ("K"=w379:dbl, "b"=w378:dbl, "X^2"=w377:dbl)
        n285 = Build Array(w407, w408, w409, w399, w398) -> (w406:dbl[])
        n286 = Build Array("泵滴定数1", "泵滴定数2", "泵滴定数3", "泵滴定数4", "泵滴定数5") -> (w405:dbl[])
        n287 = Build Array("启用1", "启用2", "启用3", "启用4", "启用5") -> (w392:bool[])
        n288 = case shown="\"多项式\"" "模型" {
          tunnel: w379 -> [w411 w414]
          tunnel: w378 -> [w410 w415]
          tunnel: w377 -> [_ w413]
          frame "线性", Default {
            "K" <- w411
            "b" <- w410
          }
          frame "多项式" {
            n289 = Build Array(w415, w414, w413) -> (→"多项式系数":dbl[])
          }
        }
        n290 = call "线性公式CODMn用.vi"("标液浓度"=w406, "监测浓度"=w405, "启用"=w392, "method"=w404, "模型"="模型", "精度"=6) -> ("拟合方程"=w385:string, "r^2"=→"r^2":dbl, "slope"=w383:dbl, "intercept"=w384:dbl, "XY图"=→"XY图":cluster{"X Values":dbl[], "Y Values":dbl[]}[], "Polynomial Coefficients"=w400:dbl[])  [unwired: 8 in]
        "拟合公式" <- w385
        n291 = feedback-in #1(w385) -> ()
        n292 = feedback #1(w385) -> (w386:string)
        n293 = Not Equal?(x=w385, y=w386) -> (x != y?=w382:bool)
        n294 = case shown="真" w382 {
          tunnel: w400 -> [_ w422]
          tunnel: w384 -> [_ w423]
          tunnel: w383 -> [_ w424]
          frame False {
          }
          frame True {
            # "当公式发生改变时赋值到右侧公式"
            n295 = local read "模型"() -> (w425:enum32{"线性", "多项式"})
            n296 = case shown="\"多项式\"" w425 {
              tunnel: [w430 w432] -> w418
              tunnel: w424 -> [w430 _]
              tunnel: w423 -> [w429 _]
              tunnel: [w429 w433] -> w419
              tunnel: w422 -> [_ w434]
              tunnel: [0.0 ("数值") w431] -> w417
              frame "线性", Default {
              }
              frame "多项式" {
                # "B,K,X^2"
                n297 = Index Array(array=w434) -> (element #1=w433:dbl, element #2=w432:dbl, element #3=w431:dbl)  [unwired: 3 in]
              }
            }
            n298 = global read "CODMn断电保存全局变量.vi" "CODMn仪器参数"() -> (w421:T7)
            n299 = local read "r^2"() -> (w416:dbl)
            n300 = Bundle By Name(cluster=cluster{"K":dbl, "b":dbl, "X^2":dbl} {"K"=0.0, "b"=0.0, "X^2"=0.0} ("方程系数"), "K"=w418, "b"=w419, "X^2"=w417) -> (w426:cluster{"K":dbl, "b":dbl, "X^2":dbl})
            n301 = Bundle By Name(cluster=w421, "曲线截距"=w419, "曲线斜率"=w418, "二次多项式系数"=w417, "线性相关系数"=w416) -> (w420:T7)
            n302 = global write "CODMn断电保存全局变量.vi" "CODMn仪器参数"(w420) -> ()
            n303 = local write "方程系数"(w426) -> ()
          }
        }
      }
    }
    n304 = flat-sequence {
      frame #0 {
        # "测量数据区"
        n305 = global read "COD内部交互全局.vi" "data"() -> (w445:T8)
        n306 = global read "CODMn断电保存全局变量.vi" "测量数据区"() -> (w439:T9)
        n307 = global read "COD测量模式全局.vi" "测量模式"() -> (w441:string)
        "测量模式(显示)" <- w441
        n308 = Unbundle By Name(w445) -> ("时间"=w444:timestamp, "检测值"=w443:sgl, "数据标识"=w442:string)
        n309 = case shown="\"水样测试\"" w441 {
          tunnel: w439 -> [w460 w465 w470 w475 w480 w485 w490 w495]
          tunnel: [w460 w464 w466 w474 w479 w484 w486 w494] -> w440
          tunnel: w444 -> [_ w463 w469 w473 w478 w483 w489 w493]
          tunnel: w443 -> [_ w462 w468 w472 w477 w482 w488 w492]
          tunnel: w442 -> [_ w461 w467 w471 w476 w481 w487 w491]
          frame "", Default {
          }
          frame "水样测试" {
            n310 = Bundle By Name(cluster=w465, "水样数据时间"=w463, "水样实测值"=w462, "水样数据标识"=w461) -> (w464:T9)
          }
          frame "标样核查" {
            n311 = Bundle By Name(cluster=w470, "跨度核查数据时间"=w469, "跨度核查实测值"=w468, "跨度核查数据标识"=w467) -> (w466:T9)
          }
          frame "零点核查" {
            n312 = Bundle By Name(cluster=w475, "零点核查数据时间"=w473, "零点核查实测值"=w472, "零点核查数据标识"=w471) -> (w474:T9)
          }
          frame "加标回收" {
            n313 = Bundle By Name(cluster=w480, "加标回收数据时间"=w478, "加标回收实测值"=w477, "加标回收数据标识"=w476) -> (w479:T9)
          }
          frame "平行样" {
            n314 = Bundle By Name(cluster=w485, "平行样数据时间"=w483, "平行样实测值"=w482, "平行样数据标识"=w481) -> (w484:T9)
          }
          frame "校零" {
            n315 = Bundle By Name(cluster=w490, "空白数据时间"=w489, "空白实测值"=w488, "空白数据标识"=w487) -> (w486:T9)
          }
          frame "校标" {
            n316 = Bundle By Name(cluster=w495, "标样数据时间"=w493, "标样实测值"=w492, "标样数据标识"=w491) -> (w494:T9)
          }
        }
        n317 = Unbundle By Name(w439) -> ("水样实测值"=w436:sgl)
        n318 = feedback-in #2(w439) -> ()
        n319 = feedback #2(w439) -> (w438:T9)
        n320 = Unbundle By Name(w438) -> ("水样实测值"=w437:sgl)
        n321 = Not Equal?(x=w436, y=w437) -> (x != y?=w435:bool)
        n322 = case shown="真" w435 {
          frame False {
          }
          frame True {
            # "水样值发送改变存储本地"
            n323 = global read "COD内部交互全局.vi" "配置文件ini"() -> (w446:string)
            n324 = call <vilib>:"Application Directory.vi"() -> ("Application Directory"=w459:path)
            n325 = Build Path(base path=w459, name or relative path=w446) -> (appended path=w458:path)
            n326 = call <vilib>:"Open Config Data.vi"("configuration file path"=w458) -> ("error out"=w454:errorcluster, "refnum"=w457:T3)  [unwired: 8 in, 1 out]
            n327 = vi-ref "斯坦道CODMn.lvlib:CODMn断电保存全局变量.vi"() -> (w456:refnum<vi>)
            n328 = call <userlib>:"Write Panel to INI__ogtk.vi"("error in (no error)"=w454, "VI ref"=w456, "refnum"=w457) -> ("error out"=w453:errorcluster, "refnum out"=w455:T3)  [unwired: 7 in]
            n329 = call <vilib>:"Close Config Data.vi"("error in (no error)"=w453, "refnum"=w455) -> ("error out"=w448:errorcluster, "file path"=w447:path)  [unwired: 8 in]
            n330 = Open/Create/Replace File(file path (use dialog)=w447, error in=w448) -> (refnum out=w451:refnum<file>, error out=w452:errorcluster)  [unwired: 4 in, 1 out]
            n331 = Flush File(refnum=w451, error in=w452) -> (refnum out=w450:refnum<file>, error out=w449:errorcluster)
            n332 = Close File(refnum=w450, error in=w449) -> ()  [unwired: 2 out]
          }
        }
        n333 = global write "CODMn断电保存全局变量.vi" "测量数据区"(w440) -> ()
      }
    }
    n334 = flat-sequence {
      frame #0 {
        # "公式读取显示（只在读取公式的时候改变一次）"
        n335 = global read "COD内部交互全局.vi" "读取公式显示"() -> (w232:bool)
        n336 = case shown="真" w232 {
          frame False {
          }
          frame True {
            n337 = global write "COD内部交互全局.vi" "读取公式显示"(FALSE ("读取参数显示")) -> ()
            n338 = global read "COD内部交互全局.vi" "读取公式"() -> (w242:u16[])
            n339 = Array Subset(array=w242, index=10 ("索引"), length=84 ("长度")) -> (w237:u16[])
            n340 = One Button Dialog(message="公式读取成功！" ("消息")) -> ()  [unwired: 1 in, 1 out]
            n341 = local read "测量模式(公式)"() -> (w240:u16)
            n342 = call "浮点CDAB转换COD.vi"("数组"=w237) -> ("数组 2"=w238:sgl[])  [unwired: 10 in]
            n343 = Array To Cluster(array=w238) -> (cluster=w241:T10)
            n344 = case shown="1" w240 {
              tunnel: [cluster{"X":dbl, "b":dbl, "X^2":dbl} {"X"=999.0, "b"=999.0, "X^2"=999.0} ("方程系数") w245 w264 w283 w302 w321 w340 w359] -> w239
              tunnel: w241 -> [_ w244 w263 w282 w301 w320 w339 w358]
              frame 0, Default {
              }
              frame 1 {
                n345 = local read "量程选择"() -> (w247:enum16{"低量程", "高量程", "0-2量程"})
                n346 = case shown="\"低量程\", 默认" w247 {
                  tunnel: w244 -> [w254 w258 w262]
                  tunnel: [w253 w257 w261] -> w250
                  tunnel: [w252 w256 w260] -> w249
                  tunnel: [w251 w255 w259] -> w248
                  frame "低量程", Default {
                    n347 = Unbundle By Name(w254) -> ("数组 2[0]"=w253:sgl, "数组 2[1]"=w252:sgl, "数组 2[2]"=w251:sgl)
                  }
                  frame "高量程" {
                    n348 = Unbundle By Name(w258) -> ("数组 2[3]"=w257:sgl, "数组 2[4]"=w256:sgl, "数组 2[5]"=w255:sgl)
                  }
                  frame "0-2量程" {
                    n349 = Unbundle By Name(w262) -> ("数组 2[6]"=w261:sgl, "数组 2[7]"=w260:sgl, "数组 2[8]"=w259:sgl)
                  }
                }
                n350 = Bundle By Name(cluster=cluster{"X":dbl, "b":dbl, "X^2":dbl} {"X"=0.0, "b"=0.0, "X^2"=0.0} ("方程系数"), "X"=w250, "b"=w249, "X^2"=w248) -> (w245:cluster{"X":dbl, "b":dbl, "X^2":dbl})
              }
              frame 2 {
                n351 = local read "量程选择"() -> (w266:enum16{"低量程", "高量程", "0-2量程"})
                n352 = case shown="\"高量程\"" w266 {
                  tunnel: w263 -> [w273 w277 w281]
                  tunnel: [w272 w276 w280] -> w269
                  tunnel: [w271 w275 w279] -> w268
                  tunnel: [w270 w274 w278] -> w267
                  frame "低量程", Default {
                    n353 = Unbundle By Name(w273) -> ("数组 2[6]"=w272:sgl, "数组 2[7]"=w271:sgl, "数组 2[8]"=w270:sgl)
                  }
                  frame "高量程" {
                    n354 = Unbundle By Name(w277) -> ("数组 2[9]"=w276:sgl, "数组 2[10]"=w275:sgl, "数组 2[11]"=w274:sgl)
                  }
                  frame "0-2量程" {
                    n355 = Unbundle By Name(w281) -> ("数组 2[6]"=w280:sgl, "数组 2[7]"=w279:sgl, "数组 2[8]"=w278:sgl)
                  }
                }
                n356 = Bundle By Name(cluster=cluster{"X":dbl, "b":dbl, "X^2":dbl} {"X"=0.0, "b"=0.0, "X^2"=0.0} ("方程系数"), "X"=w269, "b"=w268, "X^2"=w267) -> (w264:cluster{"X":dbl, "b":dbl, "X^2":dbl})
              }
              frame 3 {
                n357 = local read "量程选择"() -> (w285:enum16{"低量程", "高量程", "0-2量程"})
                n358 = case shown="\"高量程\"" w285 {
                  tunnel: w282 -> [w292 w296 w300]
                  tunnel: [w291 w295 w299] -> w288
                  tunnel: [w290 w294 w298] -> w287
                  tunnel: [w289 w293 w297] -> w286
                  frame "低量程", Default {
                    n359 = Unbundle By Name(w292) -> ("数组 2[12]"=w291:sgl, "数组 2[13]"=w290:sgl, "数组 2[14]"=w289:sgl)
                  }
                  frame "高量程" {
                    n360 = Unbundle By Name(w296) -> ("数组 2[15]"=w295:sgl, "数组 2[16]"=w294:sgl, "数组 2[17]"=w293:sgl)
                  }
                  frame "0-2量程" {
                    n361 = Unbundle By Name(w300) -> ("数组 2[6]"=w299:sgl, "数组 2[7]"=w298:sgl, "数组 2[8]"=w297:sgl)
                  }
                }
                n362 = Bundle By Name(cluster=cluster{"X":dbl, "b":dbl, "X^2":dbl} {"X"=0.0, "b"=0.0, "X^2"=0.0} ("方程系数"), "X"=w288, "b"=w287, "X^2"=w286) -> (w283:cluster{"X":dbl, "b":dbl, "X^2":dbl})
              }
              frame 4 {
                n363 = local read "量程选择"() -> (w304:enum16{"低量程", "高量程", "0-2量程"})
                n364 = case shown="\"高量程\"" w304 {
                  tunnel: w301 -> [w311 w315 w319]
                  tunnel: [w310 w314 w318] -> w307
                  tunnel: [w309 w313 w317] -> w306
                  tunnel: [w308 w312 w316] -> w305
                  frame "低量程", Default {
                    n365 = Unbundle By Name(w311) -> ("数组 2[18]"=w310:sgl, "数组 2[19]"=w309:sgl, "数组 2[20]"=w308:sgl)
                  }
                  frame "高量程" {
                    n366 = Unbundle By Name(w315) -> ("数组 2[21]"=w314:sgl, "数组 2[22]"=w313:sgl, "数组 2[23]"=w312:sgl)
                  }
                  frame "0-2量程" {
                    n367 = Unbundle By Name(w319) -> ("数组 2[6]"=w318:sgl, "数组 2[7]"=w317:sgl, "数组 2[8]"=w316:sgl)
                  }
                }
                n368 = Bundle By Name(cluster=cluster{"X":dbl, "b":dbl, "X^2":dbl} {"X"=0.0, "b"=0.0, "X^2"=0.0} ("方程系数"), "X"=w307, "b"=w306, "X^2"=w305) -> (w302:cluster{"X":dbl, "b":dbl, "X^2":dbl})
              }
              frame 5 {
                n369 = local read "量程选择"() -> (w323:enum16{"低量程", "高量程", "0-2量程"})
                n370 = case shown="\"高量程\"" w323 {
                  tunnel: w320 -> [w330 w334 w338]
                  tunnel: [w329 w333 w337] -> w326
                  tunnel: [w328 w332 w336] -> w325
                  tunnel: [w327 w331 w335] -> w324
                  frame "低量程", Default {
                    n371 = Unbundle By Name(w330) -> ("数组 2[24]"=w329:sgl, "数组 2[25]"=w328:sgl, "数组 2[26]"=w327:sgl)
                  }
                  frame "高量程" {
                    n372 = Unbundle By Name(w334) -> ("数组 2[27]"=w333:sgl, "数组 2[28]"=w332:sgl, "数组 2[29]"=w331:sgl)
                  }
                  frame "0-2量程" {
                    n373 = Unbundle By Name(w338) -> ("数组 2[6]"=w337:sgl, "数组 2[7]"=w336:sgl, "数组 2[8]"=w335:sgl)
                  }
                }
                n374 = Bundle By Name(cluster=cluster{"X":dbl, "b":dbl, "X^2":dbl} {"X"=0.0, "b"=0.0, "X^2"=0.0} ("方程系数"), "X"=w326, "b"=w325, "X^2"=w324) -> (w321:cluster{"X":dbl, "b":dbl, "X^2":dbl})
              }
              frame 6 {
                n375 = local read "量程选择"() -> (w342:enum16{"低量程", "高量程", "0-2量程"})
                n376 = case shown="\"高量程\"" w342 {
                  tunnel: w339 -> [w349 w353 w357]
                  tunnel: [w348 w352 w356] -> w345
                  tunnel: [w347 w351 w355] -> w344
                  tunnel: [w346 w350 w354] -> w343
                  frame "低量程", Default {
                    n377 = Unbundle By Name(w349) -> ("数组 2[30]"=w348:sgl, "数组 2[31]"=w347:sgl, "数组 2[32]"=w346:sgl)
                  }
                  frame "高量程" {
                    n378 = Unbundle By Name(w353) -> ("数组 2[33]"=w352:sgl, "数组 2[34]"=w351:sgl, "数组 2[35]"=w350:sgl)
                  }
                  frame "0-2量程" {
                    n379 = Unbundle By Name(w357) -> ("数组 2[6]"=w356:sgl, "数组 2[7]"=w355:sgl, "数组 2[8]"=w354:sgl)
                  }
                }
                n380 = Bundle By Name(cluster=cluster{"X":dbl, "b":dbl, "X^2":dbl} {"X"=0.0, "b"=0.0, "X^2"=0.0} ("方程系数"), "X"=w345, "b"=w344, "X^2"=w343) -> (w340:cluster{"X":dbl, "b":dbl, "X^2":dbl})
              }
              frame 7 {
                n381 = local read "量程选择"() -> (w361:enum16{"低量程", "高量程", "0-2量程"})
                n382 = case shown="\"高量程\"" w361 {
                  tunnel: w358 -> [w368 w372 w376]
                  tunnel: [w367 w371 w375] -> w364
                  tunnel: [w366 w370 w374] -> w363
                  tunnel: [w365 w369 w373] -> w362
                  frame "低量程", Default {
                    n383 = Unbundle By Name(w368) -> ("数组 2[36]"=w367:sgl, "数组 2[37]"=w366:sgl, "数组 2[38]"=w365:sgl)
                  }
                  frame "高量程" {
                    n384 = Unbundle By Name(w372) -> ("数组 2[39]"=w371:sgl, "数组 2[40]"=w370:sgl, "数组 2[41]"=w369:sgl)
                  }
                  frame "0-2量程" {
                    n385 = Unbundle By Name(w376) -> ("数组 2[6]"=w375:sgl, "数组 2[7]"=w374:sgl, "数组 2[8]"=w373:sgl)
                  }
                }
                n386 = Bundle By Name(cluster=cluster{"X":dbl, "b":dbl, "X^2":dbl} {"X"=0.0, "b"=0.0, "X^2"=0.0} ("方程系数"), "X"=w364, "b"=w363, "X^2"=w362) -> (w359:cluster{"X":dbl, "b":dbl, "X^2":dbl})
              }
            }
            n387 = local write "方程系数"(w239) -> ()
          }
        }
      }
    }
    n388 = Wait (ms)(milliseconds to wait=u32 1000 ("等待时间（毫秒）")) -> ()  [unwired: 1 out]
  }
  n389 = vi-ref "斯坦道CODMn.lvlib:待机状态数据存储写入和切换量程(子VI).vi"() -> (w36:refnum<vi>)
  n390 = vi-ref "斯坦道CODMn.lvlib:定时启动 (子VI).vi"() -> (w19:refnum<vi>)
  n391 = vi-ref "斯坦道CODMn.lvlib:日志报警状态存储 (子VI).vi"() -> (w18:refnum<vi>)
  n392 = vi-ref "斯坦道CODMn.lvlib:高锰酸钾-ORP滴定曲线(子VI).vi"() -> (w1:refnum<vi>)
  n393 = while {
    stop <- FALSE stop-if-true
    # "相差60秒自动校时"
    n394 = global read "运行时序全局变量.vi" "多列列表框"() -> (w557:i32)
    n395 = local read "仪器时间"() -> (w564:timestamp)
    n396 = local read "系统时间"() -> (w565:timestamp)
    n397 = Wait (ms)(milliseconds to wait=u32 1000 ("等待时间（毫秒）")) -> ()  [unwired: 1 out]
    n398 = Build Array(w564) -> (w563:timestamp[])
    n399 = Build Array(w565) -> (w582:timestamp[])
    n400 = Equal?(x=w557, y=u16 5) -> (x = y?=w559:bool)
    n401 = call <vilib>:"Boolean Crossing PtByPt.vi"("direction"=enum16{"either", "false-true", "true-false"}."false-true", "input"=w559) -> ("crossing"=w556:bool)  [unwired: 1 in]
    n402 = call "DateToHex.vi"("DATE"=w563) -> ("数组"=w576:u16[])  [unwired: 10 in]
    n403 = call "DateToHex.vi"("DATE"=w582) -> ("数组"=w581:u16[])  [unwired: 10 in]
    n404 = case shown="真" w556 {
      frame False {
      }
      frame True {
        # "校准结束后自动更新曲线泵滴定数"
        n405 = global read "COD测量模式全局.vi" "测量模式"() -> (w583:string)
        n406 = global read "COD内部交互全局.vi" "高锰酸钾"() -> (w586:dbl)
        n407 = Equal?(x=w583, y="校标") -> (x = y?=w585:bool)
        n408 = case shown="真" w585 {
          tunnel: w586 -> [_ w588]
          frame False {
          }
          frame True {
            n409 = global read "COD内部交互全局.vi" "当前校准"() -> (w587:i32)
            n410 = case shown="5" w587 {
              tunnel: w588 -> [w589 w590 w591 w592 w593]
              frame 1, Default {
                n411 = local write "泵滴定数1"(w589) -> ()
              }
              frame 2 {
                n412 = local write "泵滴定数2"(w590) -> ()
              }
              frame 3 {
                n413 = local write "泵滴定数3"(w591) -> ()
              }
              frame 4 {
                n414 = local write "泵滴定数4"(w592) -> ()
              }
              frame 5 {
                n415 = local write "泵滴定数5"(w593) -> ()
              }
            }
          }
        }
      }
    }
    n416 = Index Array(array=w576, index=2 ("索引")) -> (element=w578:u16)
    n417 = Index Array(array=w581, index=2 ("索引")) -> (element=w579:u16)
    n418 = Split Number(x=w578) -> (hi(x)=w572:u8)  [unwired: 1 out]
    n419 = Split Number(x=w579) -> (hi(x)=w575:u8)  [unwired: 1 out]
    n420 = To Byte Integer(number=w572) -> (8bit integer=w571:i8)
    n421 = To Byte Integer(number=w575) -> (8bit integer=w574:i8)
    n422 = Subtract(x=w571, y=w574) -> (x-y=w573:i8)
    n423 = Absolute Value(x=w573) -> (abs(x)=w570:i8)
    n424 = local read "通讯状态"() -> (w567:bool)
    n425 = Greater Or Equal?(x=w570, y=i8 60) -> (x >= y?=w568:bool)
    n426 = And(x=w568, y=w567) -> (x .and. y?=w566:bool)
    n427 = case shown="真" w566 {
      frame False {
      }
      frame True {
        # "相差60秒时间自动校准"
        n428 = flat-sequence {
          frame #0 {
            n429 = property on="时间校准" class="Bool (严格)"("Val(Sgnl)"=TRUE ("值(信号)")) -> ()  [unwired: 2 in, 2 out]
          }
          frame #1 {
            n430 = Wait (ms)(milliseconds to wait=u32 500 ("等待时间（毫秒）")) -> ()  [unwired: 1 out]
          }
          frame #2 {
            n431 = property on="时间校准" class="Bool (严格)"("Val(Sgnl)"=FALSE ("值(信号)")) -> ()  [unwired: 2 in, 2 out]
          }
        }
      }
    }
  }
  n432 = property class="VI"(reference=w19, error in=errorcluster {"status"=FALSE, "code"=0, "source"=""} ("错误输出")) -> ("Name"=w20:string)  [unwired: 2 out]
  n433 = property class="VI"(reference=w18, error in=errorcluster {"status"=FALSE, "code"=0, "source"=""} ("错误输出")) -> ("Name"=w17:string)  [unwired: 2 out]
  n434 = property class="VI"(reference=w1, error in=errorcluster {"status"=FALSE, "code"=0, "source"=""} ("错误输出")) -> ("Name"=w2:string)  [unwired: 2 out]
  n435 = Open VI Reference(type specifier VI Refnum (for type only)=refnum<vi> refnum, vi path=w20, options=128 ("选项")) -> (vi reference=w22:refnum<vi>, error out=w24:errorcluster)  [unwired: 3 in]
  n436 = property class="VI"(reference=w36, error in=errorcluster {"status"=FALSE, "code"=0, "source"=""} ("错误输出")) -> ("Name"=w35:string)  [unwired: 2 out]
  n437 = call-by-ref "?"(reference=w22, error in=w24) -> (reference out=w26:refnum<vi>, error out=w25:errorcluster)  [unwired: 12 in]
  n438 = Open VI Reference(type specifier VI Refnum (for type only)=refnum<vi> refnum, vi path=w17, options=128 ("选项")) -> (vi reference=w15:refnum<vi>, error out=w13:errorcluster)  [unwired: 3 in]
  n439 = Open VI Reference(type specifier VI Refnum (for type only)=refnum<vi> refnum, vi path=w2, options=128 ("选项")) -> (vi reference=w4:refnum<vi>, error out=w6:errorcluster)  [unwired: 3 in]
  n440 = call-by-ref "?"(reference=w15, error in=w13) -> (reference out=w11:refnum<vi>, error out=w12:errorcluster)  [unwired: 12 in]
  n441 = Close Reference(reference=w26, error in (no error)=w25) -> ()  [unwired: 1 out]
  n442 = call-by-ref "?"(reference=w4, error in=w6) -> (reference out=w8:refnum<vi>, error out=w7:errorcluster)  [unwired: 12 in]
  n443 = Open VI Reference(type specifier VI Refnum (for type only)=refnum<vi> refnum, vi path=w35, options=128 ("选项")) -> (vi reference=w33:refnum<vi>, error out=w31:errorcluster)  [unwired: 3 in]
  n444 = Close Reference(reference=w11, error in (no error)=w12) -> ()  [unwired: 1 out]
  n445 = call-by-ref "?"(reference=w33, error in=w31) -> (reference out=w29:refnum<vi>, error out=w30:errorcluster)  [unwired: 12 in]
  n446 = Close Reference(reference=w8, error in (no error)=w7) -> ()  [unwired: 1 out]
  n447 = Close Reference(reference=w29, error in (no error)=w30) -> ()  [unwired: 1 out]
  n448 = Obtain Queue(name (unnamed)="CODMn" ("名称（未命名）"), element data type=cluster{"命令":string} {"命令"="启用模块"} ("元素")) -> (queue out=w48:refnum<queue>, error out=w47:errorcluster)  [unwired: 3 in, 1 out]
  n449 = vi-ref "CODMn通讯.vi"() -> (w38:refnum<vi>)
  n450 = while {
    tunnel: w48 -> [w606]
    tunnel: w47 -> [w605]
    tunnel: w39 -> [_]
    stop <- FALSE stop-if-true
    # "主循环界面显示"
    n451 = flat-sequence {
      frame #0 {
        # "A，B，K"
        # "CODMn读取状态"
        n452 = global read "COD内部交互全局.vi" "ORP、时间"() -> (w738:u16[])
        n453 = To Word Integer(number=w738) -> (16bit integer=w759:i16[])
        n454 = Split 1D Array(array=w759, index=3 ("索引")) -> (first subarray=w740:i16[], second subarray=w758:i16[])
        n455 = Index Array(array=w740) -> (element #1=w744:i16, element #2=w743:i16, element #3=w742:i16)  [unwired: 3 in]
        n456 = Index Array(array=w758) -> (element #1=w753:i16, element #2=w757:i16, element #3=w756:i16, element #4=w755:i16)  [unwired: 4 in]
        n457 = To Single Precision Float(number=w755) -> (single precision float=w746:sgl)
        n458 = Build Array(w744, w743, w742) -> (w741:i16[])
        n459 = To Single Precision Float(number=w753) -> (single precision float=w752:sgl)
        n460 = To Single Precision Float(number=w757) -> (single precision float=w751:sgl)
        n461 = To Single Precision Float(number=w756) -> (single precision float=w747:sgl)
        n462 = call "HexToDate.vi"("数组"=w741) -> ("DATE"=w745:timestamp[])  [unwired: 10 in]
        n463 = Number To Decimal String(number=w751) -> (decimal integer string=→"ORP-A":string)  [unwired: 1 in]
        n464 = Number To Decimal String(number=w747) -> (decimal integer string=→"ORP-B":string)  [unwired: 1 in]
        n465 = Number To Decimal String(number=w746) -> (decimal integer string=→"ORP-K":string)  [unwired: 1 in]
        n466 = Divide(x=w752, y=sgl 100.0) -> (x/y=→"COD浓度（mg/L)":sgl)
        n467 = Index Array(array=w745) -> (element=w739:timestamp)  [unwired: 1 in]
        n468 = Format Date/Time String(seconds (now)=w739) -> (date/time string=→"数据时间":string)  [unwired: 2 in]
      }
    }
    n469 = flat-sequence {
      frame #0 {
        # "测量状态显示"
        n470 = global read "COD内部交互全局.vi" "测量状态"() -> (w650:u16[])
        n471 = To Word Integer(number=w650) -> (16bit integer=w661:i16[])
        n472 = Index Array(array=w661, index #1=0 ("索引"), index #4=3 ("索引"), index #14=13 ("索引"), index #15=14 ("索引"), index #21=20 ("索引"), index #32=31 ("索引")) -> (element #1=w666:i16, element #2=w665:i16, element #3=w664:i16, element #4=→"CODMn工作状态":i16, element #5=→"模式（受控）":i16, element #6=→"进样管":i16, element #7=→"高锰酸钾":i16, element #8=→"草酸钠":i16, element #9=→"硫酸":i16, element #10=w660:i16, element #11=w681:i16, element #12=w656:i16, element #13=→"报警数字":i16, element #14=w687:i16, element #15=w672:i16, element #16=→"多列列表框":i16, element #21=w648:i16, element #33=→"分":i16, element #34=→"秒":i16)  [unwired: 28 in, 15 out]
        n473 = global write "COD内部交互全局.vi" "基本量程存储数据用"(w648) -> ()
        n474 = Build Array(w666, w665, w664) -> (w667:i16[])
        n475 = To Single Precision Float(number=w660) -> (single precision float=→"ORP显示":sgl)
        n476 = Number To Decimal String(number=w648) -> (decimal integer string=→"基本量程(显示)":string)  [unwired: 1 in]
        n477 = Equal?(x=w656, y=u16 1) -> (x = y?=→"排液标记":bool)
        n478 = Equal?(x=w656, y=u16 2) -> (x = y?=→"断电排液标记":bool)
        n479 = Divide(x=w681, y=u16 10) -> (x/y=→"温度":dbl)
        n480 = Divide(x=w687, y=u16 1000) -> (x/y=→"零点滴定值":dbl)
        n481 = Divide(x=w672, y=u16 1000) -> (x/y=→"标度滴定值":dbl)
        n482 = call "HexToDate.vi"("数组"=w667) -> ("DATE"=w662:timestamp[])  [unwired: 10 in]
        n483 = Index Array(array=w662) -> (element=→"仪器时间":timestamp)  [unwired: 1 in]
      }
    }
    n484 = flat-sequence {
      frame #0 {
        # "报警状态显示"
        n485 = local read "报警数字"() -> (w691:i16)
        n486 = Equal?(x=w691, y=u16 1) -> (x = y?=w702:bool)
        "ORP故障" <- w702
        n487 = Equal?(x=w691, y=u16 2) -> (x = y?=w701:bool)
        "温控器故障" <- w701
        n488 = Equal?(x=w691, y=u16 3) -> (x = y?=w700:bool)
        "加热故障" <- w700
        n489 = Equal?(x=w691, y=u16 6) -> (x = y?=w697:bool)
        "测量错误" <- w697
        n490 = Equal?(x=w691, y=u16 8) -> (x = y?=w696:bool)
        "校零错误" <- w696
        n491 = Equal?(x=w691, y=u16 7) -> (x = y?=w695:bool)
        "校标错误" <- w695
        n492 = Equal?(x=w691, y=u16 9) -> (x = y?=w694:bool)
        "进水样超量程" <- w694
        n493 = Equal?(x=w691, y=u16 10) -> (x = y?=w693:bool)
        "排液故障" <- w693
        n494 = Equal?(x=w691, y=u16 4) -> (x = y?=w699:bool)
        "高锰酸钾报警" <- w699
        n495 = Equal?(x=w691, y=u16 5) -> (x = y?=w698:bool)
        "草酸钠报警" <- w698
        n496 = Compound Arithmetic op=OR ("复合运算")(w702, w701, w700, w699, w698, w697, w695, w696, w694, w693) -> (→"故障标记":bool)
        n497 = Bundle By Name(cluster=T11 {"ORP故障"=FALSE, "温控器故障"=FALSE, "加热故障"=FALSE, "高锰酸钾报警"=FALSE, "草酸钠报警"=FALSE, "测量错误"=FALSE, "校零错误"=FALSE, "校标错误"=FALSE, " 进水样超量程"=FALSE, "排液阀故障"=FALSE} ("报警簇"), "ORP故障"=w702, "温控器故障"=w701, "加热故障"=w700, "高锰酸钾报警"=w699, "草酸钠报警"=w698, "测量错误"=w697, "校零错误"=w696, "校标错误"=w695, "进水样超量程"=w694, "排液阀故障"=w693) -> (w690:T11)
        n498 = global write "COD内部交互全局.vi" "报警簇"(w690) -> ()
      }
    }
    n499 = flat-sequence {
      frame #0 {
        # "CODMn读取状态"
        n500 = global read "COD内部交互全局.vi" "温度"() -> (w735:bool[])
        n501 = global read "COD内部交互全局.vi" "M输出点"() -> (w734:bool[])
        n502 = Index Array(array=w735) -> (element=→"加热":bool)  [unwired: 1 in]
        n503 = Index Array(array=w734) -> (element #1=→"搅拌":bool, element #4=→"进水样":bool, element #5=→"进蒸馏水":bool, element #6=→"进标液":bool, element #7=→"进零点核查样":bool, element #8=→"进加标回收样":bool, element #9=→"进高锰酸钾":bool, element #10=→"进草酸钠":bool, element #11=→"进硫酸":bool)  [unwired: 11 in, 2 out]
      }
    }
    n504 = flat-sequence {
      frame #0 {
        # "工作状态显示"
        n505 = local read "CODMn工作状态"() -> (w616:T1)
        n506 = case shown="\"标样校准\"" w616 {
          tunnel: [_ u16 0 ("y") u16 1 ("y") u16 2 ("y") u16 3 ("y") u16 4 ("y") u16 6 ("y") _ u16 7 ("y") u16 8 ("y") u16 5 ("y")] -> w615
          frame "空闲", Default {
          }
          frame "水样测试" {
          }
          frame "标样核查" {
          }
          frame "零点核查" {
          }
          frame "跨度核查" {
          }
          frame "空白测试" {
          }
          frame "平行样测试" {
          }
          frame "质控样" {
          }
          frame "空白校准" {
          }
          frame "标样校准" {
          }
          frame "加标回收" {
          }
        }
        n507 = Equal?(x=w616, y=u16 8) -> (x = y?=→"校零标记":bool)
        n508 = Equal?(x=w616, y=u16 4) -> (x = y?=→"跨度核查标记":bool)
        n509 = Equal?(x=w616, y=u16 0) -> (x = y?=→"待机":bool)
        n510 = Equal?(x=w616, y=u16 3) -> (x = y?=→"零点核查标记":bool)
        n511 = Equal?(x=w616, y=u16 7) -> (x = y?=→"质控样测量":bool)
        n512 = Equal?(x=w616, y=u16 1) -> (x = y?=→"水样测量":bool)
        n513 = Equal?(x=w616, y=u16 2) -> (x = y?=→"标样核查标记":bool)
        n514 = Equal?(x=w616, y=u16 6) -> (x = y?=→"平行样测量":bool)
        n515 = Equal?(x=w616, y=u16 9) -> (x = y?=→"校标标记":bool)
        n516 = Equal?(x=w616, y=u16 5) -> (x = y?=→"空白测试标记":bool)
        n517 = Equal?(x=w616, y=u16 10) -> (x = y?=→"加标回收测量":bool)
        n518 = global write "COD内部交互全局.vi" "测量模式数字"(w615) -> ()
      }
    }
    n519 = Get Date/Time In Seconds() -> (seconds since 1Jan1904=→"系统时间":timestamp)
    n520 = First Call?() -> (First Call?: T/F=w604:bool)
    n521 = Wait (ms)(milliseconds to wait=u32 1000 ("等待时间（毫秒）")) -> ()  [unwired: 1 out]
    n522 = case shown="真" w604 {
      tunnel: w606 -> [w715 w720]
      tunnel: w605 -> [w714 w719]
      tunnel: [w715 w718] -> w602
      tunnel: [w714 w717] -> w601
      frame False {
      }
      frame True {
        n523 = Bundle By Name(cluster=cluster{"命令":string} {"命令"=""} ("元素"), "命令"="CODMn读取参数" ("名称（未命名）")) -> (w723:cluster{"命令":string})
        n524 = Enqueue Element(queue=w720, element=w723, timeout in ms (-1)=1000 ("超时毫秒(-1)"), error in (no error)=w719) -> (queue out=w718:refnum<queue>, error out=w717:errorcluster)  [unwired: 1 out]
      }
    }
    n525 = Get Queue Status(queue=w602, error in (no error)=w601) -> (queue out=w598:refnum<queue>, error out=w597:errorcluster, # elements in queue=w600:i32)  [unwired: 1 in, 5 out]
    n526 = Equal To 0?(x=w600) -> (x = 0?=w599:bool)
    n527 = case shown="真" w599 {
      tunnel: w598 -> [_ w610]
      tunnel: w597 -> [_ w609]
      frame False {
      }
      frame True {
        n528 = Bundle By Name(cluster=cluster{"命令":string} {"命令"=""} ("元素"), "命令"="CODMn读取" ("名称（未命名）")) -> (w612:cluster{"命令":string})
        n529 = Enqueue Element(queue=w610, element=w612, timeout in ms (-1)=1000 ("超时毫秒(-1)"), error in (no error)=w609) -> ()  [unwired: 3 out]
      }
    }
  }
  n530 = while {
    tunnel: w48 -> [w762]
    tunnel: w47 -> [w761]
    stop <- FALSE stop-if-true
    # "主线事件"
    n531 = event shown="[6] \"保存\": 鼠标按下" {
      selector: _ -> [_ _ _ _ _ _ _ _ _ _ _ _ _ _ _ _ _ _ _ _ _ _ _ _ _ _ _ _ _ _ _ _ _]
      dyn-events: _ -> [_ _ _ _ _ _ _ _ _ _ _ _ _ _ _ _ _ _ _ _ _ _ _ _ _ _ _ _ _ _ _ _ _]
      timeout: _ -> [_ _ _ _ _ _ _ _ _ _ _ _ _ _ _ _ _ _ _ _ _ _ _ _ _ _ _ _ _ _ _ _ _]
      tunnel: w762 -> [_ _ _ _ _ w819 _ _ _ _ _ _ _ _ _ _ _ _ _ _ _ _ _ _ _ w1470 _ _ _ _ w1717 w1724 _]
      tunnel: w761 -> [_ _ _ _ _ w818 _ _ _ _ _ _ _ _ _ _ _ _ _ _ _ _ _ _ _ w1469 _ _ _ _ w1716 w1723 _]
      event "单步启动": Mouse Down {
        n532 = event-data() -> ()  [unwired: 1 in, 8 out]
        n533 = call "CODMn手动控制框.vi"() -> ()  [unwired: 12 in]
      }
      event "启动": Mouse Down {
        n534 = event-data() -> ()  [unwired: 1 in, 8 out]
        n535 = flat-sequence {
          tunnel: [w765] -> w764
          tunnel: w764 -> [w771]
          frame #0 {
            n536 = call "启动测量模式选择对话框.vi"() -> ("启动选择 2"=w765:u16)  [unwired: 11 in]
            "启动选择 2" <- w765
          }
          frame #1 {
            n537 = case shown="9, 默认" w771 {
              tunnel: [u16 4608 ("address") u16 4608 ("address") u16 4608 ("address") u16 4608 ("address") u16 4608 ("address") u16 4608 ("address") u16 4608 ("address") u16 4608 ("address") u16 4608 ("address") u16 4608 ("address")] -> w767
              tunnel: [u16 1 ("address") u16 2 ("address") u16 3 ("address") u16 4 ("address") u16 5 ("address") u16 7 ("address") u16 6 ("address") u16 8 ("address") u16 9 ("address") u16 0 ("address")] -> w772
              frame 0 {
              }
              frame 1 {
              }
              frame 2 {
              }
              frame 3 {
              }
              frame 4 {
              }
              frame 5 {
              }
              frame 6 {
              }
              frame 7 {
              }
              frame 8 {
              }
              frame 9, Default {
              }
            }
            n538 = Not Equal?(x=w771, y=u16 9) -> (x != y?=w769:bool)
            n539 = global write "CODMN外部API.vi" "手动启动CODMn"(w769) -> ()
            n540 = Insert Into Array(array=u16[] [] ("values"), index=0 ("索引"), new element=w772) -> (w766:u16[])
            n541 = call "CODMnMB_api.vi"("STEP"=enum16{"open", "read", "write", "close"}."write", "values"=w766, "starting address"=w767) -> ()  [unwired: 6 in, 3 out]
          }
        }
      }
      event "停止": Value Change {
        n542 = event-data() -> ()  [unwired: 1 in, 6 out]
        n543 = Two Button Dialog(message="确认是否停止？" ("消息"), 1:"否" ("F按钮名称（“取消”）"), 2:"是" ("T按钮名称（“确定”）")) -> (T button?=w797:bool)
        n544 = case shown="真" w797 {
          frame False {
          }
          frame True {
            n545 = call "CODMnMB_api.vi"("STEP"=enum16{"open", "read", "write", "close"}."write", "values"=u16[] [11], "starting address"=u16 4608) -> ()  [unwired: 6 in, 3 out]
          }
        }
      }
      event "手动控制": Value Change {
        n546 = event-data() -> ()  [unwired: 1 in, 6 out]
        n547 = call "数字密码键盘.vi"() -> ("NewNumber"=w802:sgl)  [unwired: 1 in]
        n548 = Equal?(x=w802, y=8.0) -> (x = y?=w803:bool)
        n549 = case shown="假" w803 {
          frame False {
            n550 = call "窗口弹出对话框(子VI).vi"("消息"="密码错误") -> ()  [unwired: 10 in, 1 out]
          }
          frame True {
          }
        }
      }
      event "锁定按钮": Mouse Down {
        n551 = event-data() -> ("CtlRef"=w808:refnum<vi>)  [unwired: 1 in, 7 out]
        n552 = property class="Bool (严格)"(reference=w808) -> ("Value"=w807:bool)  [unwired: 1 in, 2 out]
        n553 = case shown="真" w807 {
          selector: w807 -> [w809 _]
          tunnel: [w809 w810] -> w806
          frame False {
          }
          frame True {
            n554 = call "数字密码键盘.vi"() -> ("NewNumber"=w811:sgl)  [unwired: 1 in]
            n555 = Equal?(x=w811, y=8.0) -> (x = y?=w810:bool)
            n556 = case shown="假" w810 {
              selector: w810 -> [w814 _]
              frame False {
                n557 = local write "锁定按钮"(w814) -> ()
                n558 = One Button Dialog(message="密码错误!" ("消息")) -> ()  [unwired: 1 in, 1 out]
              }
              frame True {
                n559 = One Button Dialog(message="解锁成功!" ("消息")) -> ()  [unwired: 1 in, 1 out]
              }
            }
          }
        }
        "x = y?" <- w806
      }
      event "参数配置": Value Change {
        (unwired) u16 20 ("number of holding registers")
        (unwired) u16 4272 ("starting address")
        n560 = event-data() -> ()  [unwired: 1 in, 6 out]
        n561 = global read "COD内部交互全局.vi" "配置文件ini"() -> (w816:string)
        n562 = property on="窗格" class="Pane"("Origin"=T2 {"Horizontal"=0, "Vertical"=650} ("原点")) -> ()  [unwired: 2 in, 2 out]
        n563 = call <vilib>:"Application Directory.vi"() -> ("Application Directory"=w823:path)
        n564 = Build Path(base path=w823, name or relative path=w816) -> (appended path=w824:path)
        n565 = Bundle By Name(cluster=cluster{"命令":string} {"命令"=""} ("元素"), "命令"="CODMn读取参数" ("名称（未命名）")) -> (w820:cluster{"命令":string})
        n566 = call <vilib>:"Open Config Data.vi"("configuration file path"=w824) -> ("error out"=w828:errorcluster, "refnum"=w825:T3)  [unwired: 8 in, 1 out]
        n567 = Enqueue Element(queue=w819, element=w820, error in (no error)=w818) -> ()  [unwired: 1 in, 3 out]
        n568 = vi-ref "斯坦道CODMn.lvlib:CODMn断电保存全局变量.vi"() -> (w826:refnum<vi>)
        n569 = call <userlib>:"Read Panel from INI__ogtk.vi"("error in (no error)"=w828, "VI ref"=w826, "refnum"=w825) -> ("error out"=w829:errorcluster, "refnum out"=w827:T3)  [unwired: 7 in]
        n570 = call <vilib>:"Close Config Data.vi"("error in (no error)"=w829, "refnum"=w827) -> ("error out"=w830:errorcluster, "file path"=w831:path)  [unwired: 8 in]
        n571 = Open/Create/Replace File(file path (use dialog)=w831, error in=w830) -> (error out=w817:errorcluster)  [unwired: 4 in, 2 out]
        n572 = call <vilib>:"Clear Errors.vi"("error in (no error)"=w817) -> ()  [unwired: 5 in, 2 out]
      }
      event "保存": Mouse Down {
        n573 = event-data() -> ()  [unwired: 1 in, 8 out]
        n574 = local read "通讯状态"() -> (w833:bool)
        n575 = Two Button Dialog(message="确定保存参数，保存参数将会替换原有参数！" ("消息")) -> (T button?=w835:bool)  [unwired: 2 in]
        n576 = case shown="真" w835 {
          tunnel: w833 -> [_ w836]
          frame False {
          }
          frame True {
            n577 = case shown="真" w836 {
              frame False {
                n578 = One Button Dialog(message="保存失败，当前无通讯！" ("消息")) -> ()  [unwired: 1 in, 1 out]
              }
              frame True {
                n579 = One Button Dialog(message="参数保存成功！" ("消息")) -> ()  [unwired: 1 in, 1 out]
                n580 = Build Array("采水泵进样时间/s:", "采水泵润洗时间/s:", "采水泵沉淀时间/s:", "采水泵排液时间/s:") -> (w839:i32[])
                n581 = call "CODMnMB_api.vi"("STEP"=enum16{"open", "read", "write", "close"}."write", "values"="保存参数", "starting address"=u16 4272) -> ("error out"=w845:errorcluster)  [unwired: 6 in, 2 out]
                n582 = call "CODMnMB_api.vi"("STEP"=enum16{"open", "read", "write", "close"}."write", "Error in"=w845, "values"=w839, "starting address"=u16 5596) -> ()  [unwired: 5 in, 3 out]
              }
            }
          }
        }
      }
      event "常规版/认证版": Value Change {
        n583 = event-data() -> ()  [unwired: 1 in, 6 out]
        n584 = flat-sequence {
          frame #0 {
            n585 = global write "CODMn断电保存全局变量.vi" "常规版/认证版"("常规版/认证版") -> ()
          }
          frame #1 {
            n586 = global read "COD内部交互全局.vi" "配置文件ini"() -> (w851:string)
            n587 = call <vilib>:"Application Directory.vi"() -> ("Application Directory"=w864:path)
            n588 = Build Path(base path=w864, name or relative path=w851) -> (appended path=w863:path)
            n589 = call <vilib>:"Open Config Data.vi"("configuration file path"=w863) -> ("error out"=w859:errorcluster, "refnum"=w862:T3)  [unwired: 8 in, 1 out]
            n590 = vi-ref "斯坦道CODMn.lvlib:CODMn断电保存全局变量.vi"() -> (w861:refnum<vi>)
            n591 = call <userlib>:"Write Panel to INI__ogtk.vi"("error in (no error)"=w859, "VI ref"=w861, "refnum"=w862) -> ("error out"=w858:errorcluster, "refnum out"=w860:T3)  [unwired: 7 in]
            n592 = call <vilib>:"Close Config Data.vi"("error in (no error)"=w858, "refnum"=w860) -> ("error out"=w853:errorcluster, "file path"=w852:path)  [unwired: 8 in]
            n593 = Open/Create/Replace File(file path (use dialog)=w852, error in=w853) -> (refnum out=w856:refnum<file>, error out=w857:errorcluster)  [unwired: 4 in, 1 out]
            n594 = Flush File(refnum=w856, error in=w857) -> (refnum out=w855:refnum<file>, error out=w854:errorcluster)
            n595 = Close File(refnum=w855, error in=w854) -> ()  [unwired: 2 out]
          }
        }
      }
      event "校准配置": Value Change {
        n596 = event-data() -> ()  [unwired: 1 in, 6 out]
        n597 = global read "COD内部交互全局.vi" "配置文件ini"() -> (w865:string)
        n598 = property on="窗格" class="Pane"("Origin"=T2 {"Horizontal"=0, "Vertical"=1300} ("原点")) -> ()  [unwired: 2 in, 2 out]
        n599 = call <vilib>:"Application Directory.vi"() -> ("Application Directory"=w915:path)
        n600 = Build Path(base path=w915, name or relative path=w865) -> (appended path=w914:path)
        n601 = call <vilib>:"Open Config Data.vi"("configuration file path"=w914) -> ("error out"=w884:errorcluster, "refnum"=w885:T3)  [unwired: 8 in, 1 out]
        n602 = call-poly <vilib>:"Read Key.vi"("section"="CODMn模型选择" ("key"), "error in (no error)"=w884, "key"="线性和多项式", "refnum"=w885) -> ("error out"=w881:errorcluster, "value"=w883:i32, "refnum out"=w882:T3)  [unwired: 4 in, 1 out]
        n603 = local write "模型"(w883) -> ()
        n604 = call-poly <vilib>:"Read Key.vi"("section"="标线选择", "error in (no error)"=w881, "key"="选用水样", "refnum"=w882) -> ("error out"=w879:errorcluster, "value"=w866:i32, "refnum out"=w880:T3)  [unwired: 4 in, 1 out]
        n605 = local write "选用水样"(w866) -> ()
        n606 = case shown="0, 默认" w866 {
          tunnel: ["葡萄糖标线" ("section") "草酸钠标线" ("section")] -> w890
          frame 0, Default {
          }
          frame 1 {
          }
        }
        n607 = local read "量程选择"() -> (w891:enum16{"低量程", "高量程", "0-2量程"})
        n608 = case shown="\"0-2量程\"" w891 {
          tunnel: ["低量程" "高量程" "0-2量程"] -> w889
          frame "低量程", Default {
          }
          frame "高量程" {
          }
          frame "0-2量程" {
          }
        }
        n609 = Concatenate Strings(w890, w889) -> (w888:string)
        n610 = call-poly <vilib>:"Read Key.vi"("section"=w888, "error in (no error)"=w879, "key"="浓度1", "refnum"=w880) -> ("error out"=w919:errorcluster, "value"=w917:dbl, "refnum out"=w918:T3)  [unwired: 4 in, 1 out]
        n611 = local write "浓度1"(w917) -> ()
        n612 = call-poly <vilib>:"Read Key.vi"("section"=w888, "error in (no error)"=w919, "key"="浓度2", "refnum"=w918) -> ("error out"=w933:errorcluster, "value"=w920:dbl, "refnum out"=w932:T3)  [unwired: 4 in, 1 out]
        n613 = local write "浓度2"(w920) -> ()
        n614 = call-poly <vilib>:"Read Key.vi"("section"=w888, "error in (no error)"=w933, "key"="浓度3", "refnum"=w932) -> ("error out"=w934:errorcluster, "value"=w922:dbl, "refnum out"=w931:T3)  [unwired: 4 in, 1 out]
        n615 = local write "浓度3"(w922) -> ()
        n616 = call-poly <vilib>:"Read Key.vi"("section"=w888, "error in (no error)"=w934, "key"="泵滴定数1", "refnum"=w931) -> ("error out"=w935:errorcluster, "value"=w924:dbl, "refnum out"=w930:T3)  [unwired: 4 in, 1 out]
        n617 = local write "泵滴定数1"(w924) -> ()
        n618 = call-poly <vilib>:"Read Key.vi"("section"=w888, "error in (no error)"=w935, "key"="泵滴定数2", "refnum"=w930) -> ("error out"=w929:errorcluster, "value"=w927:dbl, "refnum out"=w936:T3)  [unwired: 4 in, 1 out]
        n619 = local write "泵滴定数2"(w927) -> ()
        n620 = call-poly <vilib>:"Read Key.vi"("section"=w888, "error in (no error)"=w929, "key"="泵滴定数3", "refnum"=w936) -> ("error out"=w941:errorcluster, "value"=w940:dbl, "refnum out"=w937:T3)  [unwired: 4 in, 1 out]
        n621 = local write "泵滴定数3"(w940) -> ()
        n622 = call-poly <vilib>:"Read Key.vi"("section"=w888, "error in (no error)"=w941, "key"="浓度4", "refnum"=w937) -> ("error out"=w942:errorcluster, "value"=w872:dbl, "refnum out"=w938:T3)  [unwired: 4 in, 1 out]
        n623 = local write "浓度4"(w872) -> ()
        n624 = call-poly <vilib>:"Read Key.vi"("section"=w888, "error in (no error)"=w942, "key"="浓度5", "refnum"=w938) -> ("error out"=w877:errorcluster, "value"=w871:dbl, "refnum out"=w878:T3)  [unwired: 4 in, 1 out]
        n625 = local write "浓度5"(w871) -> ()
        n626 = call-poly <vilib>:"Read Key.vi"("section"=w888, "error in (no error)"=w877, "key"="泵滴定数4", "refnum"=w878) -> ("error out"=w943:errorcluster, "value"=w870:dbl, "refnum out"=w939:T3)  [unwired: 4 in, 1 out]
        n627 = local write "泵滴定数4"(w870) -> ()
        n628 = call-poly <vilib>:"Read Key.vi"("section"=w888, "error in (no error)"=w943, "key"="泵滴定数5", "refnum"=w939) -> ("error out"=w875:errorcluster, "value"=w869:dbl, "refnum out"=w876:T3)  [unwired: 4 in, 1 out]
        n629 = local write "泵滴定数5"(w869) -> ()
        n630 = call-poly <vilib>:"Read Key.vi"("section"=w888, "error in (no error)"=w875, "key"="当前选用的校准", "refnum"=w876) -> ("error out"=w910:errorcluster, "value"=w912:i32, "refnum out"=w911:T3)  [unwired: 4 in, 1 out]
        n631 = local write "当前校准"(w912) -> ()
        n632 = call-poly <vilib>:"Read Key.vi"("section"=w888, "error in (no error)"=w910, "key"="启用1", "refnum"=w911) -> ("error out"=w907:errorcluster, "value"=w896:bool, "refnum out"=w908:T3)  [unwired: 4 in, 1 out]
        n633 = local write "启用1"(w896) -> ()
        n634 = call-poly <vilib>:"Read Key.vi"("section"=w888, "error in (no error)"=w907, "key"="启用2", "refnum"=w908) -> ("error out"=w905:errorcluster, "value"=w895:bool, "refnum out"=w906:T3)  [unwired: 4 in, 1 out]
        n635 = local write "启用2"(w895) -> ()
        n636 = call-poly <vilib>:"Read Key.vi"("section"=w888, "error in (no error)"=w905, "key"="启用3", "refnum"=w906) -> ("error out"=w903:errorcluster, "value"=w894:bool, "refnum out"=w904:T3)  [unwired: 4 in, 1 out]
        n637 = local write "启用3"(w894) -> ()
        n638 = call-poly <vilib>:"Read Key.vi"("section"=w888, "error in (no error)"=w903, "key"="启用4", "refnum"=w904) -> ("error out"=w901:errorcluster, "value"=w868:bool, "refnum out"=w902:T3)  [unwired: 4 in, 1 out]
        n639 = local write "启用4"(w868) -> ()
        n640 = call-poly <vilib>:"Read Key.vi"("section"=w888, "error in (no error)"=w901, "key"="启用5", "refnum"=w902) -> ("error out"=w873:errorcluster, "value"=w867:bool, "refnum out"=w874:T3)  [unwired: 4 in, 1 out]
        n641 = local write "启用5"(w867) -> ()
        n642 = call <vilib>:"Close Config Data.vi"("error in (no error)"=w873, "refnum"=w874) -> ()  [unwired: 8 in, 2 out]
      }
      event "选用水样": Value Change {
        (unwired) "浓度6" ("key")
        n643 = event-data() -> ()  [unwired: 1 in, 6 out]
        n644 = global read "COD内部交互全局.vi" "配置文件ini"() -> (w954:string)
        n645 = local read "量程选择"() -> (w968:enum16{"低量程", "高量程", "0-2量程"})
        n646 = property on="窗格" class="Pane"("Origin"=T2 {"Horizontal"=0, "Vertical"=1300} ("原点")) -> ()  [unwired: 2 in, 2 out]
        n647 = case shown="\"葡萄糖\", 默认" "选用水样" {
          tunnel: ["葡萄糖标线" ("section") "草酸钠标线" ("section")] -> w970
          frame "葡萄糖", Default {
          }
          frame "草酸钠" {
          }
        }
        n648 = call <vilib>:"Application Directory.vi"() -> ("Application Directory"=w993:path)
        n649 = case shown="\"0-2量程\"" w968 {
          tunnel: ["低量程" "高量程" "0-2量程"] -> w969
          frame "低量程", Default {
          }
          frame "高量程" {
          }
          frame "0-2量程" {
          }
        }
        n650 = Build Path(base path=w993, name or relative path=w954) -> (appended path=w992:path)
        n651 = Concatenate Strings(w970, w969) -> (w967:string)
        n652 = call <vilib>:"Open Config Data.vi"("configuration file path"=w992) -> ("error out"=w994:errorcluster, "refnum"=w995:T3)  [unwired: 8 in, 1 out]
        n653 = call-poly <vilib>:"Read Key.vi"("section"=w967, "error in (no error)"=w994, "key"="浓度1", "refnum"=w995) -> ("error out"=w999:errorcluster, "value"=w997:dbl, "refnum out"=w998:T3)  [unwired: 4 in, 1 out]
        n654 = local write "浓度1"(w997) -> ()
        n655 = call-poly <vilib>:"Read Key.vi"("section"=w967, "error in (no error)"=w999, "key"="浓度2", "refnum"=w998) -> ("error out"=w1013:errorcluster, "value"=w1000:dbl, "refnum out"=w1012:T3)  [unwired: 4 in, 1 out]
        n656 = local write "浓度2"(w1000) -> ()
        n657 = call-poly <vilib>:"Read Key.vi"("section"=w967, "error in (no error)"=w1013, "key"="浓度3", "refnum"=w1012) -> ("error out"=w1014:errorcluster, "value"=w1002:dbl, "refnum out"=w1011:T3)  [unwired: 4 in, 1 out]
        n658 = local write "浓度3"(w1002) -> ()
        n659 = call-poly <vilib>:"Read Key.vi"("section"=w967, "error in (no error)"=w1014, "key"="泵滴定数1", "refnum"=w1011) -> ("error out"=w1015:errorcluster, "value"=w1004:dbl, "refnum out"=w1010:T3)  [unwired: 4 in, 1 out]
        n660 = local write "泵滴定数1"(w1004) -> ()
        n661 = call-poly <vilib>:"Read Key.vi"("section"=w967, "error in (no error)"=w1015, "key"="泵滴定数2", "refnum"=w1010) -> ("error out"=w1009:errorcluster, "value"=w1007:dbl, "refnum out"=w1016:T3)  [unwired: 4 in, 1 out]
        n662 = local write "泵滴定数2"(w1007) -> ()
        n663 = call-poly <vilib>:"Read Key.vi"("section"=w967, "error in (no error)"=w1009, "key"="泵滴定数3", "refnum"=w1016) -> ("error out"=w1021:errorcluster, "value"=w1020:dbl, "refnum out"=w1017:T3)  [unwired: 4 in, 1 out]
        n664 = local write "泵滴定数3"(w1020) -> ()
        n665 = call-poly <vilib>:"Read Key.vi"("section"=w967, "error in (no error)"=w1021, "key"="浓度4", "refnum"=w1017) -> ("error out"=w1022:errorcluster, "value"=w962:dbl, "refnum out"=w1018:T3)  [unwired: 4 in, 1 out]
        n666 = local write "浓度4"(w962) -> ()
        n667 = call-poly <vilib>:"Read Key.vi"("section"=w967, "error in (no error)"=w1022, "key"="浓度5", "refnum"=w1018) -> ("error out"=w965:errorcluster, "value"=w961:dbl, "refnum out"=w966:T3)  [unwired: 4 in, 1 out]
        n668 = local write "浓度5"(w961) -> ()
        n669 = call-poly <vilib>:"Read Key.vi"("section"=w967, "error in (no error)"=w965, "key"="泵滴定数4", "refnum"=w966) -> ("error out"=w1023:errorcluster, "value"=w960:dbl, "refnum out"=w1019:T3)  [unwired: 4 in, 1 out]
        n670 = local write "泵滴定数4"(w960) -> ()
        n671 = call-poly <vilib>:"Read Key.vi"("section"=w967, "error in (no error)"=w1023, "key"="泵滴定数5", "refnum"=w1019) -> ("error out"=w963:errorcluster, "value"=w959:dbl, "refnum out"=w964:T3)  [unwired: 4 in, 1 out]
        n672 = local write "泵滴定数5"(w959) -> ()
        n673 = call-poly <vilib>:"Read Key.vi"("section"=w967, "error in (no error)"=w963, "key"="当前选用的校准", "refnum"=w964) -> ("error out"=w988:errorcluster, "value"=w990:i32, "refnum out"=w989:T3)  [unwired: 4 in, 1 out]
        n674 = local write "当前校准"(w990) -> ()
        n675 = call-poly <vilib>:"Read Key.vi"("section"=w967, "error in (no error)"=w988, "key"="启用1", "refnum"=w989) -> ("error out"=w985:errorcluster, "value"=w974:bool, "refnum out"=w986:T3)  [unwired: 4 in, 1 out]
        n676 = local write "启用1"(w974) -> ()
        n677 = call-poly <vilib>:"Read Key.vi"("section"=w967, "error in (no error)"=w985, "key"="启用2", "refnum"=w986) -> ("error out"=w983:errorcluster, "value"=w973:bool, "refnum out"=w984:T3)  [unwired: 4 in, 1 out]
        n678 = local write "启用2"(w973) -> ()
        n679 = call-poly <vilib>:"Read Key.vi"("section"=w967, "error in (no error)"=w983, "key"="启用3", "refnum"=w984) -> ("error out"=w981:errorcluster, "value"=w972:bool, "refnum out"=w982:T3)  [unwired: 4 in, 1 out]
        n680 = local write "启用3"(w972) -> ()
        n681 = call-poly <vilib>:"Read Key.vi"("section"=w967, "error in (no error)"=w981, "key"="启用4", "refnum"=w982) -> ("error out"=w979:errorcluster, "value"=w956:bool, "refnum out"=w980:T3)  [unwired: 4 in, 1 out]
        n682 = local write "启用4"(w956) -> ()
        n683 = call-poly <vilib>:"Read Key.vi"("section"=w967, "error in (no error)"=w979, "key"="启用5", "refnum"=w980) -> ("error out"=w957:errorcluster, "value"=w955:bool, "refnum out"=w958:T3)  [unwired: 4 in, 1 out]
        n684 = local write "启用5"(w955) -> ()
        n685 = call <vilib>:"Close Config Data.vi"("error in (no error)"=w957, "refnum"=w958) -> ()  [unwired: 8 in, 2 out]
      }
      event "量程选择": Value Change {
        n686 = event-data() -> ()  [unwired: 1 in, 6 out]
        n687 = global read "COD内部交互全局.vi" "配置文件ini"() -> (w1034:string)
        n688 = local read "选用水样"() -> (w1051:enum16{"葡萄糖", "草酸钠"})
        n689 = property on="窗格" class="Pane"("Origin"=T2 {"Horizontal"=0, "Vertical"=1300} ("原点")) -> ()  [unwired: 2 in, 2 out]
        n690 = call <vilib>:"Application Directory.vi"() -> ("Application Directory"=w1073:path)
        n691 = case shown="\"葡萄糖\", 默认" w1051 {
          tunnel: ["葡萄糖标线" ("section") "草酸钠标线" ("section")] -> w1050
          frame "葡萄糖", Default {
          }
          frame "草酸钠" {
          }
        }
        n692 = Build Path(base path=w1073, name or relative path=w1034) -> (appended path=w1072:path)
        n693 = case shown="\"0-2量程\"" "量程选择" {
          tunnel: ["低量程" "高量程" "0-2量程"] -> w1047
          frame "低量程", Default {
          }
          frame "高量程" {
          }
          frame "0-2量程" {
          }
        }
        n694 = Concatenate Strings(w1050, w1047) -> (w1049:string)
        n695 = call <vilib>:"Open Config Data.vi"("configuration file path"=w1072) -> ("error out"=w1074:errorcluster, "refnum"=w1075:T3)  [unwired: 8 in, 1 out]
        n696 = call-poly <vilib>:"Read Key.vi"("section"=w1049, "error in (no error)"=w1074, "key"="浓度1", "refnum"=w1075) -> ("error out"=w1079:errorcluster, "value"=w1077:dbl, "refnum out"=w1078:T3)  [unwired: 4 in, 1 out]
        n697 = local write "浓度1"(w1077) -> ()
        n698 = call-poly <vilib>:"Read Key.vi"("section"=w1049, "error in (no error)"=w1079, "key"="浓度2", "refnum"=w1078) -> ("error out"=w1093:errorcluster, "value"=w1080:dbl, "refnum out"=w1092:T3)  [unwired: 4 in, 1 out]
        n699 = local write "浓度2"(w1080) -> ()
        n700 = call-poly <vilib>:"Read Key.vi"("section"=w1049, "error in (no error)"=w1093, "key"="浓度3", "refnum"=w1092) -> ("error out"=w1094:errorcluster, "value"=w1082:dbl, "refnum out"=w1091:T3)  [unwired: 4 in, 1 out]
        n701 = local write "浓度3"(w1082) -> ()
        n702 = call-poly <vilib>:"Read Key.vi"("section"=w1049, "error in (no error)"=w1094, "key"="泵滴定数1", "refnum"=w1091) -> ("error out"=w1095:errorcluster, "value"=w1084:dbl, "refnum out"=w1090:T3)  [unwired: 4 in, 1 out]
        n703 = local write "泵滴定数1"(w1084) -> ()
        n704 = call-poly <vilib>:"Read Key.vi"("section"=w1049, "error in (no error)"=w1095, "key"="泵滴定数2", "refnum"=w1090) -> ("error out"=w1089:errorcluster, "value"=w1087:dbl, "refnum out"=w1096:T3)  [unwired: 4 in, 1 out]
        n705 = local write "泵滴定数2"(w1087) -> ()
        n706 = call-poly <vilib>:"Read Key.vi"("section"=w1049, "error in (no error)"=w1089, "key"="泵滴定数3", "refnum"=w1096) -> ("error out"=w1101:errorcluster, "value"=w1100:dbl, "refnum out"=w1097:T3)  [unwired: 4 in, 1 out]
        n707 = local write "泵滴定数3"(w1100) -> ()
        n708 = call-poly <vilib>:"Read Key.vi"("section"=w1049, "error in (no error)"=w1101, "key"="浓度4", "refnum"=w1097) -> ("error out"=w1102:errorcluster, "value"=w1038:dbl, "refnum out"=w1098:T3)  [unwired: 4 in, 1 out]
        n709 = local write "浓度4"(w1038) -> ()
        n710 = call-poly <vilib>:"Read Key.vi"("section"=w1049, "error in (no error)"=w1102, "key"="浓度5", "refnum"=w1098) -> ("error out"=w1045:errorcluster, "value"=w1037:dbl, "refnum out"=w1046:T3)  [unwired: 4 in, 1 out]
        n711 = local write "浓度5"(w1037) -> ()
        n712 = call-poly <vilib>:"Read Key.vi"("section"=w1049, "error in (no error)"=w1045, "key"="泵滴定数4", "refnum"=w1046) -> ("error out"=w1103:errorcluster, "value"=w1036:dbl, "refnum out"=w1099:T3)  [unwired: 4 in, 1 out]
        n713 = local write "泵滴定数4"(w1036) -> ()
        n714 = call-poly <vilib>:"Read Key.vi"("section"=w1049, "error in (no error)"=w1103, "key"="泵滴定数5", "refnum"=w1099) -> ("error out"=w1043:errorcluster, "value"=w1035:dbl, "refnum out"=w1044:T3)  [unwired: 4 in, 1 out]
        n715 = local write "泵滴定数5"(w1035) -> ()
        n716 = call-poly <vilib>:"Read Key.vi"("section"=w1049, "error in (no error)"=w1043, "key"="当前选用的校准", "refnum"=w1044) -> ("error out"=w1068:errorcluster, "value"=w1070:i32, "refnum out"=w1069:T3)  [unwired: 4 in, 1 out]
        n717 = local write "当前校准"(w1070) -> ()
        n718 = call-poly <vilib>:"Read Key.vi"("section"=w1049, "error in (no error)"=w1068, "key"="启用1", "refnum"=w1069) -> ("error out"=w1065:errorcluster, "value"=w1054:bool, "refnum out"=w1066:T3)  [unwired: 4 in, 1 out]
        n719 = local write "启用1"(w1054) -> ()
        n720 = call-poly <vilib>:"Read Key.vi"("section"=w1049, "error in (no error)"=w1065, "key"="启用2", "refnum"=w1066) -> ("error out"=w1063:errorcluster, "value"=w1053:bool, "refnum out"=w1064:T3)  [unwired: 4 in, 1 out]
        n721 = local write "启用2"(w1053) -> ()
        n722 = call-poly <vilib>:"Read Key.vi"("section"=w1049, "error in (no error)"=w1063, "key"="启用3", "refnum"=w1064) -> ("error out"=w1061:errorcluster, "value"=w1052:bool, "refnum out"=w1062:T3)  [unwired: 4 in, 1 out]
        n723 = local write "启用3"(w1052) -> ()
        n724 = call-poly <vilib>:"Read Key.vi"("section"=w1049, "error in (no error)"=w1061, "key"="启用4", "refnum"=w1062) -> ("error out"=w1059:errorcluster, "value"=w1040:bool, "refnum out"=w1060:T3)  [unwired: 4 in, 1 out]
        n725 = local write "启用4"(w1040) -> ()
        n726 = call-poly <vilib>:"Read Key.vi"("section"=w1049, "error in (no error)"=w1059, "key"="启用5", "refnum"=w1060) -> ("error out"=w1041:errorcluster, "value"=w1039:bool, "refnum out"=w1042:T3)  [unwired: 4 in, 1 out]
        n727 = local write "启用5"(w1039) -> ()
        n728 = call <vilib>:"Close Config Data.vi"("error in (no error)"=w1041, "refnum"=w1042) -> ()  [unwired: 8 in, 2 out]
      }
      event "返回": Value Change {
        w1128 = "CODMn" ("section")
        n729 = event-data() -> ()  [unwired: 1 in, 6 out]
        n730 = global read "COD内部交互全局.vi" "配置文件ini"() -> (w1114:string)
        n731 = property on="窗格" class="Pane"("Origin"=T2 {"Horizontal"=0, "Vertical"=0} ("原点")) -> ()  [unwired: 2 in, 2 out]
        n732 = call <vilib>:"Application Directory.vi"() -> ("Application Directory"=w1180:path)
        n733 = Build Path(base path=w1180, name or relative path=w1114) -> (appended path=w1179:path)
        n734 = call <vilib>:"Open Config Data.vi"("configuration file path"=w1179) -> ("error out"=w1177:errorcluster, "refnum"=w1178:T3)  [unwired: 8 in, 1 out]
        n735 = local read "浓度1"() -> (w1175:dbl)
        n736 = call-poly <vilib>:"Write Key.vi"("section"=w1128, "error in (no error)"=w1177, "value"=w1175, "key"="浓度1", "refnum"=w1178) -> ("error out"=w1174:errorcluster, "refnum out"=w1173:T3)  [unwired: 4 in, 1 out]
        n737 = local read "浓度2"() -> (w1159:dbl)
        n738 = call-poly <vilib>:"Write Key.vi"("section"=w1128, "error in (no error)"=w1174, "value"=w1159, "key"="浓度2", "refnum"=w1173) -> ("error out"=w1172:errorcluster, "refnum out"=w1171:T3)  [unwired: 4 in, 1 out]
        n739 = local read "浓度3"() -> (w1155:dbl)
        n740 = local read "泵滴定数1"() -> (w1153:dbl)
        n741 = call-poly <vilib>:"Write Key.vi"("section"=w1128, "error in (no error)"=w1172, "value"=w1155, "key"="浓度3", "refnum"=w1171) -> ("error out"=w1170:errorcluster, "refnum out"=w1169:T3)  [unwired: 4 in, 1 out]
        n742 = local read "泵滴定数2"() -> (w1151:dbl)
        n743 = call-poly <vilib>:"Write Key.vi"("section"=w1128, "error in (no error)"=w1170, "value"=w1153, "key"="泵滴定数1", "refnum"=w1169) -> ("error out"=w1168:errorcluster, "refnum out"=w1167:T3)  [unwired: 4 in, 1 out]
        n744 = local read "泵滴定数3"() -> (w1149:dbl)
        n745 = call-poly <vilib>:"Write Key.vi"("section"=w1128, "error in (no error)"=w1168, "value"=w1151, "key"="泵滴定数2", "refnum"=w1167) -> ("error out"=w1166:errorcluster, "refnum out"=w1165:T3)  [unwired: 4 in, 1 out]
        n746 = call-poly <vilib>:"Write Key.vi"("section"=w1128, "error in (no error)"=w1166, "value"=w1149, "key"="泵滴定数3", "refnum"=w1165) -> ("error out"=w1164:errorcluster, "refnum out"=w1163:T3)  [unwired: 4 in, 1 out]
        n747 = local read "浓度4"() -> (w1116:dbl)
        n748 = call-poly <vilib>:"Write Key.vi"("section"=w1128, "error in (no error)"=w1164, "value"=w1116, "key"="浓度4", "refnum"=w1163) -> ("error out"=w1157:errorcluster, "refnum out"=w1158:T3)  [unwired: 4 in, 1 out]
        n749 = local read "浓度5"() -> (w1115:dbl)
        n750 = local read "泵滴定数4"() -> (w1117:dbl)
        n751 = call-poly <vilib>:"Write Key.vi"("section"=w1128, "error in (no error)"=w1157, "value"=w1115, "key"="浓度5", "refnum"=w1158) -> ("error out"=w1125:errorcluster, "refnum out"=w1126:T3)  [unwired: 4 in, 1 out]
        n752 = local read "泵滴定数5"() -> (w1118:dbl)
        n753 = call-poly <vilib>:"Write Key.vi"("section"=w1128, "error in (no error)"=w1125, "value"=w1117, "key"="泵滴定数4", "refnum"=w1126) -> ("error out"=w1162:errorcluster, "refnum out"=w1161:T3)  [unwired: 4 in, 1 out]
        n754 = call-poly <vilib>:"Write Key.vi"("section"=w1128, "error in (no error)"=w1162, "value"=w1118, "key"="泵滴定数5", "refnum"=w1161) -> ("error out"=w1123:errorcluster, "refnum out"=w1124:T3)  [unwired: 4 in, 1 out]
        n755 = local read "启用1"() -> (w1137:bool)
        n756 = call-poly <vilib>:"Write Key.vi"("section"=w1128, "error in (no error)"=w1123, "value"=w1137, "key"="启用1", "refnum"=w1124) -> ("error out"=w1133:errorcluster, "refnum out"=w1136:T3)  [unwired: 4 in, 1 out]
        n757 = local read "启用2"() -> (w1134:bool)
        n758 = call-poly <vilib>:"Write Key.vi"("section"=w1128, "error in (no error)"=w1133, "value"=w1134, "key"="启用2", "refnum"=w1136) -> ("error out"=w1144:errorcluster, "refnum out"=w1143:T3)  [unwired: 4 in, 1 out]
        n759 = local read "启用3"() -> (w1132:bool)
        n760 = call-poly <vilib>:"Write Key.vi"("section"=w1128, "error in (no error)"=w1144, "value"=w1132, "key"="启用3", "refnum"=w1143) -> ("error out"=w1142:errorcluster, "refnum out"=w1141:T3)  [unwired: 4 in, 1 out]
        n761 = local read "启用4"() -> (w1120:bool)
        n762 = call-poly <vilib>:"Write Key.vi"("section"=w1128, "error in (no error)"=w1142, "value"=w1120, "key"="启用4", "refnum"=w1141) -> ("error out"=w1140:errorcluster, "refnum out"=w1139:T3)  [unwired: 4 in, 1 out]
        n763 = local read "启用5"() -> (w1119:bool)
        n764 = call-poly <vilib>:"Write Key.vi"("section"=w1128, "error in (no error)"=w1140, "value"=w1119, "key"="启用5", "refnum"=w1139) -> ("error out"=w1121:errorcluster, "refnum out"=w1122:T3)  [unwired: 4 in, 1 out]
        n765 = call <vilib>:"Close Config Data.vi"("error in (no error)"=w1121, "refnum"=w1122) -> ()  [unwired: 8 in, 2 out]
      }
      event "关闭", "关闭 2", "关闭 3": Value Change {
        n766 = event-data() -> ()  [unwired: 1 in, 6 out]
        n767 = property on="窗格" class="Pane"("Origin"=T2 {"Horizontal"=0, "Vertical"=0} ("原点")) -> ()  [unwired: 2 in, 2 out]
      }
      event Application Instance Close {
        n768 = event-data() -> ()  [unwired: 1 in, 4 out]
      }
      event "时间校准": Value Change {
        n769 = event-data() -> ()  [unwired: 1 in, 6 out]
        n770 = Get Date/Time In Seconds() -> (seconds since 1Jan1904=w1190:timestamp)
        n771 = Build Array(w1190) -> (w1189:timestamp[])
        n772 = call "DateToHex.vi"("DATE"=w1189) -> ("数组"=w1187:u16[])  [unwired: 10 in]
        n773 = Insert Into Array(array=u16[] [1] ("values"), index=1 ("索引"), new element=w1187) -> (w1183:u16[])
        n774 = call "CODMnMB_api.vi"("STEP"=enum16{"open", "read", "write", "close"}."write", "values"=w1183, "starting address"=u16 4612) -> ("error out"=w1182:errorcluster)  [unwired: 6 in, 2 out]
        n775 = call <vilib>:"Clear Errors.vi"("error in (no error)"=w1182) -> ()  [unwired: 5 in, 2 out]
      }
      event "故障清除": Value Change {
        n776 = event-data() -> ()  [unwired: 1 in, 6 out]
        n777 = call "CODMnMB_api.vi"("STEP"=enum16{"open", "read", "write", "close"}."write", "values"=u16[] [1], "starting address"=u16 4611) -> ()  [unwired: 6 in, 3 out]
      }
      event "定时启动": Mouse Down {
        n778 = event-data() -> ()  [unwired: 1 in, 8 out]
        n779 = flat-sequence {
          frame #0 {
            n780 = global read "CODMn断电保存全局变量.vi" "定时控制"() -> (w1195:T5)
            n781 = call "周期设置.vi"("定时控制参数输入"=w1195) -> ("定时控制参数输出"=w1194:T5)  [unwired: 10 in]
            n782 = global write "CODMn断电保存全局变量.vi" "定时控制"(w1194) -> ()
          }
          frame #1 {
            n783 = global read "COD内部交互全局.vi" "配置文件ini"() -> (w1196:string)
            n784 = call <vilib>:"Application Directory.vi"() -> ("Application Directory"=w1209:path)
            n785 = Build Path(base path=w1209, name or relative path=w1196) -> (appended path=w1208:path)
            n786 = call <vilib>:"Open Config Data.vi"("configuration file path"=w1208) -> ("error out"=w1204:errorcluster, "refnum"=w1207:T3)  [unwired: 8 in, 1 out]
            n787 = vi-ref "斯坦道CODMn.lvlib:CODMn断电保存全局变量.vi"() -> (w1206:refnum<vi>)
            n788 = call <userlib>:"Write Panel to INI__ogtk.vi"("error in (no error)"=w1204, "VI ref"=w1206, "refnum"=w1207) -> ("error out"=w1203:errorcluster, "refnum out"=w1205:T3)  [unwired: 7 in]
            n789 = call <vilib>:"Close Config Data.vi"("error in (no error)"=w1203, "refnum"=w1205) -> ("error out"=w1198:errorcluster, "file path"=w1197:path)  [unwired: 8 in]
            n790 = Open/Create/Replace File(file path (use dialog)=w1197, error in=w1198) -> (refnum out=w1201:refnum<file>, error out=w1202:errorcluster)  [unwired: 4 in, 1 out]
            n791 = Flush File(refnum=w1201, error in=w1202) -> (refnum out=w1200:refnum<file>, error out=w1199:errorcluster)
            n792 = Close File(refnum=w1200, error in=w1199) -> ()  [unwired: 2 out]
          }
        }
      }
      event "仪器参数": Value Change {
        n793 = event-data() -> ()  [unwired: 1 in, 6 out]
        n794 = global read "CODMn断电保存全局变量.vi" "CODMn仪器参数"() -> (w1210:T7)
        n795 = call "仪器参数设置.vi"("仪器参数设置"=w1210) -> ("仪器参数设置输出"=w1211:T13)  [unwired: 10 in]
        n796 = Unbundle By Name(w1211) -> ("确定"=w1212:bool)
        n797 = case shown="真" w1212 {
          tunnel: w1211 -> [_ w1214]
          tunnel: w1210 -> [_ w1213]
          frame False {
          }
          frame True {
            n798 = flat-sequence {
              tunnel: w1214 -> [w1231]
              tunnel: w1213 -> [w1230]
              frame #0 {
                n799 = Unbundle By Name(w1231) -> ("测量量程"=w1229:dbl, "测量精度"=w1228:dbl, "测量间隔"=w1227:dbl, "消解温度"=w1226:dbl, "消解时长"=w1225:dbl, "空白校准时间"=w1224:timestamp, "曲线截距"=w1223:dbl, "曲线斜率"=w1222:dbl, "测量检出限"=w1221:dbl, "测量信号值"=w1220:dbl, "线性相关系数"=w1219:dbl, "二次多项式系数"=w1218:dbl, "标样校准时间"=w1217:timestamp, "单位"=w1216:u16)
                n800 = Bundle By Name(cluster=w1230, "测量量程"=w1229, "测量精度"=w1228, "测量间隔"=w1227, "消解温度"=w1226, "消解时长"=w1225, "空白校准时间"=w1224, "曲线截距"=w1223, "曲线斜率"=w1222, "测量检出限"=w1221, "测量信号值"=w1220, "线性相关系数"=w1219, "二次多项式系数"=w1218, "标样校准时间"=w1217, "单位"=w1216) -> (w1215:T7)
                n801 = global write "CODMn断电保存全局变量.vi" "CODMn仪器参数"(w1215) -> ()
              }
              frame #1 {
                n802 = global read "COD内部交互全局.vi" "配置文件ini"() -> (w1232:string)
                n803 = call <vilib>:"Application Directory.vi"() -> ("Application Directory"=w1245:path)
                n804 = Build Path(base path=w1245, name or relative path=w1232) -> (appended path=w1244:path)
                n805 = call <vilib>:"Open Config Data.vi"("configuration file path"=w1244) -> ("error out"=w1240:errorcluster, "refnum"=w1243:T3)  [unwired: 8 in, 1 out]
                n806 = vi-ref "斯坦道CODMn.lvlib:CODMn断电保存全局变量.vi"() -> (w1242:refnum<vi>)
                n807 = call <userlib>:"Write Panel to INI__ogtk.vi"("error in (no error)"=w1240, "VI ref"=w1242, "refnum"=w1243) -> ("error out"=w1239:errorcluster, "refnum out"=w1241:T3)  [unwired: 7 in]
                n808 = call <vilib>:"Close Config Data.vi"("error in (no error)"=w1239, "refnum"=w1241) -> ("error out"=w1234:errorcluster, "file path"=w1233:path)  [unwired: 8 in]
                n809 = Open/Create/Replace File(file path (use dialog)=w1233, error in=w1234) -> (refnum out=w1237:refnum<file>, error out=w1238:errorcluster)  [unwired: 4 in, 1 out]
                n810 = Flush File(refnum=w1237, error in=w1238) -> (refnum out=w1236:refnum<file>, error out=w1235:errorcluster)
                n811 = Close File(refnum=w1236, error in=w1235) -> ()  [unwired: 2 out]
              }
            }
          }
        }
      }
      event "远程自动校准浓度", "远程校准量程": Value Change {
        n812 = event-data() -> ()  [unwired: 1 in, 6 out]
        n813 = flat-sequence {
          frame #0 {
            n814 = global write "CODMn断电保存全局变量.vi" "远程校准量程"("远程校准量程") -> ()
            n815 = global write "CODMn断电保存全局变量.vi" "远程自动校准浓度"("远程自动校准浓度") -> ()
          }
          frame #1 {
            n816 = global read "COD内部交互全局.vi" "配置文件ini"() -> (w1248:string)
            n817 = call <vilib>:"Application Directory.vi"() -> ("Application Directory"=w1261:path)
            n818 = Build Path(base path=w1261, name or relative path=w1248) -> (appended path=w1260:path)
            n819 = call <vilib>:"Open Config Data.vi"("configuration file path"=w1260) -> ("error out"=w1256:errorcluster, "refnum"=w1259:T3)  [unwired: 8 in, 1 out]
            n820 = vi-ref "斯坦道CODMn.lvlib:CODMn断电保存全局变量.vi"() -> (w1258:refnum<vi>)
            n821 = call <userlib>:"Write Panel to INI__ogtk.vi"("error in (no error)"=w1256, "VI ref"=w1258, "refnum"=w1259) -> ("error out"=w1255:errorcluster, "refnum out"=w1257:T3)  [unwired: 7 in]
            n822 = call <vilib>:"Close Config Data.vi"("error in (no error)"=w1255, "refnum"=w1257) -> ("error out"=w1250:errorcluster, "file path"=w1249:path)  [unwired: 8 in]
            n823 = Open/Create/Replace File(file path (use dialog)=w1249, error in=w1250) -> (refnum out=w1253:refnum<file>, error out=w1254:errorcluster)  [unwired: 4 in, 1 out]
            n824 = Flush File(refnum=w1253, error in=w1254) -> (refnum out=w1252:refnum<file>, error out=w1251:errorcluster)
            n825 = Close File(refnum=w1252, error in=w1251) -> ()  [unwired: 2 out]
          }
        }
      }
      event "测量模式(公式)": Value Change {
        n826 = event-data() -> ()  [unwired: 1 in, 6 out]
        n827 = flat-sequence {
          frame #0 {
            n828 = global write "CODMn断电保存全局变量.vi" "测量模式(公式)"("测量模式(公式)") -> ()
          }
          frame #1 {
            n829 = global read "COD内部交互全局.vi" "配置文件ini"() -> (w1263:string)
            n830 = call <vilib>:"Application Directory.vi"() -> ("Application Directory"=w1276:path)
            n831 = Build Path(base path=w1276, name or relative path=w1263) -> (appended path=w1275:path)
            n832 = call <vilib>:"Open Config Data.vi"("configuration file path"=w1275) -> ("error out"=w1271:errorcluster, "refnum"=w1274:T3)  [unwired: 8 in, 1 out]
            n833 = vi-ref "斯坦道CODMn.lvlib:CODMn断电保存全局变量.vi"() -> (w1273:refnum<vi>)
            n834 = call <userlib>:"Write Panel to INI__ogtk.vi"("error in (no error)"=w1271, "VI ref"=w1273, "refnum"=w1274) -> ("error out"=w1270:errorcluster, "refnum out"=w1272:T3)  [unwired: 7 in]
            n835 = call <vilib>:"Close Config Data.vi"("error in (no error)"=w1270, "refnum"=w1272) -> ("error out"=w1265:errorcluster, "file path"=w1264:path)  [unwired: 8 in]
            n836 = Open/Create/Replace File(file path (use dialog)=w1264, error in=w1265) -> (refnum out=w1268:refnum<file>, error out=w1269:errorcluster)  [unwired: 4 in, 1 out]
            n837 = Flush File(refnum=w1268, error in=w1269) -> (refnum out=w1267:refnum<file>, error out=w1266:errorcluster)
            n838 = Close File(refnum=w1267, error in=w1266) -> ()  [unwired: 2 out]
          }
        }
      }
      event "跨度量程选择", "跨度液浓度", "零点核查量程选择", "零点核查浓度", "标样浓度", "标样核查量程选择": Value Change {
        n839 = event-data() -> ()  [unwired: 1 in, 6 out]
        n840 = flat-sequence {
          frame #0 {
            n841 = global write "CODMn断电保存全局变量.vi" "标样浓度"("标样浓度") -> ()
            n842 = global write "CODMn断电保存全局变量.vi" "零点核查浓度"("零点核查浓度") -> ()
            n843 = global write "CODMn断电保存全局变量.vi" "跨度液浓度"("跨度液浓度") -> ()
            n844 = global write "CODMn断电保存全局变量.vi" "CODMn跨度量程选择"("跨度量程选择") -> ()
            n845 = global write "CODMn断电保存全局变量.vi" "标样核查量程选择"("标样核查量程选择") -> ()
            n846 = global write "CODMn断电保存全局变量.vi" "零点核查量程选择"("零点核查量程选择") -> ()
          }
          frame #1 {
            n847 = global read "COD内部交互全局.vi" "配置文件ini"() -> (w1283:string)
            n848 = call <vilib>:"Application Directory.vi"() -> ("Application Directory"=w1296:path)
            n849 = Build Path(base path=w1296, name or relative path=w1283) -> (appended path=w1295:path)
            n850 = call <vilib>:"Open Config Data.vi"("configuration file path"=w1295) -> ("error out"=w1291:errorcluster, "refnum"=w1294:T3)  [unwired: 8 in, 1 out]
            n851 = vi-ref "斯坦道CODMn.lvlib:CODMn断电保存全局变量.vi"() -> (w1293:refnum<vi>)
            n852 = call <userlib>:"Write Panel to INI__ogtk.vi"("error in (no error)"=w1291, "VI ref"=w1293, "refnum"=w1294) -> ("error out"=w1290:errorcluster, "refnum out"=w1292:T3)  [unwired: 7 in]
            n853 = call <vilib>:"Close Config Data.vi"("error in (no error)"=w1290, "refnum"=w1292) -> ("error out"=w1285:errorcluster, "file path"=w1284:path)  [unwired: 8 in]
            n854 = Open/Create/Replace File(file path (use dialog)=w1284, error in=w1285) -> (refnum out=w1288:refnum<file>, error out=w1289:errorcluster)  [unwired: 4 in, 1 out]
            n855 = Flush File(refnum=w1288, error in=w1289) -> (refnum out=w1287:refnum<file>, error out=w1286:errorcluster)
            n856 = Close File(refnum=w1287, error in=w1286) -> ()  [unwired: 2 out]
          }
        }
      }
      event "校准1", "校准2", "校准3", "校准4", "校准5": Value Change {
        n857 = event-data() -> ()  [unwired: 1 in, 6 out]
        n858 = flat-sequence {
          frame #0 {
            n859 = Build Array("校准1", "校准2", "校准3", "校准4", "校准5") -> (w1299:bool[])
            n860 = for {
              tunnel: w1299 -> [w1310] mode=indexing
              i -> [w1303]
              n861 = case shown="2" w1303 {
                tunnel: ["浓度1" "浓度2" "浓度3" "浓度4" "浓度5"] -> w1306
                frame 0, Default {
                }
                frame 1 {
                }
                frame 2 {
                }
                frame 3 {
                }
                frame 4 {
                }
              }
              n862 = Multiply(x=w1306, y=100.0) -> (x*y=w1304:dbl)
              n863 = Insert Into Array(array=u16[] [] ("values"), index=0 ("索引"), new element=w1304) -> (w1307:u16[])
              n864 = case shown="真" w1310 {
                tunnel: w1307 -> [_ w1317]
                tunnel: w1303 -> [_ w1320]
                frame False {
                }
                frame True {
                  n865 = Increment(x=w1320) -> (x+1=→"当前校准":i32)
                  n866 = call "CODMnMB_api.vi"("STEP"=enum16{"open", "read", "write", "close"}."write", "values"=w1317, "starting address"=u16 4274) -> ()  [unwired: 6 in, 3 out]
                }
              }
            }
          }
          frame #1 {
            n867 = local read "当前校准"() -> (w1327:i32)
            n868 = case shown="5" w1327 {
              tunnel: [w1331 w1332 w1333 w1334 w1335] -> w1326
              frame 1, Default {
                n869 = local read "浓度1"() -> (w1331:dbl)
              }
              frame 2 {
                n870 = local read "浓度2"() -> (w1332:dbl)
              }
              frame 3 {
                n871 = local read "浓度3"() -> (w1333:dbl)
              }
              frame 4 {
                n872 = local read "浓度4"() -> (w1334:dbl)
              }
              frame 5 {
                n873 = local read "浓度5"() -> (w1335:dbl)
              }
            }
            n874 = Not Equal To 0?(x=w1326) -> (x != 0?=w1324:bool)
            n875 = case shown="真" w1324 {
              tunnel: [u16 8 ("address") u16 9 ("address")] -> w1330
              tunnel: ["校零" ("测量模式") "校标" ("测量模式")] -> w1325
              frame False {
              }
              frame True {
              }
            }
            n876 = global write "COD测量模式全局.vi" "测量模式"(w1325) -> ()
            n877 = Insert Into Array(array=u16[] [] ("values"), index=0 ("索引"), new element=w1330) -> (w1321:u16[])
            n878 = call "CODMnMB_api.vi"("STEP"=enum16{"open", "read", "write", "close"}."write", "values"=w1321, "starting address"=u16 4608 ("address")) -> ()  [unwired: 6 in, 3 out]
          }
          frame #2 {
            n879 = global read "COD内部交互全局.vi" "配置文件ini"() -> (w1340:string)
            n880 = local read "选用水样"() -> (w1343:enum16{"葡萄糖", "草酸钠"})
            n881 = local read "量程选择"() -> (w1342:enum16{"低量程", "高量程", "0-2量程"})
            n882 = call <vilib>:"Application Directory.vi"() -> ("Application Directory"=w1352:path)
            n883 = case shown="\"葡萄糖\", 默认" w1343 {
              tunnel: ["葡萄糖标线" ("section") "草酸钠标线" ("section")] -> w1344
              frame "葡萄糖", Default {
              }
              frame "草酸钠" {
              }
            }
            n884 = Build Path(base path=w1352, name or relative path=w1340) -> (appended path=w1353:path)
            n885 = case shown="\"0-2量程\"" w1342 {
              tunnel: ["低量程" "高量程" "0-2量程"] -> w1345
              frame "低量程", Default {
              }
              frame "高量程" {
              }
              frame "0-2量程" {
              }
            }
            n886 = local read "当前校准"() -> (w1348:i32)
            n887 = Concatenate Strings(w1344, w1345) -> (w1341:string)
            n888 = call <vilib>:"Open Config Data.vi"("configuration file path"=w1353) -> ("error out"=w1350:errorcluster, "refnum"=w1351:T3)  [unwired: 8 in, 1 out]
            n889 = call-poly <vilib>:"Write Key.vi"("section"=w1341, "error in (no error)"=w1350, "value"=w1348, "key"="当前选用的校准" ("section"), "refnum"=w1351) -> ("error out"=w1346:errorcluster, "refnum out"=w1347:T3)  [unwired: 4 in, 1 out]
            n890 = call <vilib>:"Close Config Data.vi"("error in (no error)"=w1346, "refnum"=w1347) -> ()  [unwired: 8 in, 2 out]
          }
        }
      }
      event "自动切换量程:", "低切高阈值:", "高切低阈值:": Value Change {
        n891 = event-data() -> ()  [unwired: 1 in, 6 out]
        n892 = flat-sequence {
          frame #0 {
            n893 = global write "CODMn断电保存全局变量.vi" "高切低阈值:"("高切低阈值:") -> ()
            n894 = global write "CODMn断电保存全局变量.vi" "自动切换量程:"("自动切换量程:") -> ()
            n895 = global write "CODMn断电保存全局变量.vi" "低切高阈值:"("低切高阈值:") -> ()
          }
          frame #1 {
            n896 = global read "COD内部交互全局.vi" "配置文件ini"() -> (w1362:string)
            n897 = call <vilib>:"Application Directory.vi"() -> ("Application Directory"=w1375:path)
            n898 = Build Path(base path=w1375, name or relative path=w1362) -> (appended path=w1374:path)
            n899 = call <vilib>:"Open Config Data.vi"("configuration file path"=w1374) -> ("error out"=w1370:errorcluster, "refnum"=w1373:T3)  [unwired: 8 in, 1 out]
            n900 = vi-ref "斯坦道CODMn.lvlib:CODMn断电保存全局变量.vi"() -> (w1372:refnum<vi>)
            n901 = call <userlib>:"Write Panel to INI__ogtk.vi"("error in (no error)"=w1370, "VI ref"=w1372, "refnum"=w1373) -> ("error out"=w1369:errorcluster, "refnum out"=w1371:T3)  [unwired: 7 in]
            n902 = call <vilib>:"Close Config Data.vi"("error in (no error)"=w1369, "refnum"=w1371) -> ("error out"=w1364:errorcluster, "file path"=w1363:path)  [unwired: 8 in]
            n903 = Open/Create/Replace File(file path (use dialog)=w1363, error in=w1364) -> (refnum out=w1367:refnum<file>, error out=w1368:errorcluster)  [unwired: 4 in, 1 out]
            n904 = Flush File(refnum=w1367, error in=w1368) -> (refnum out=w1366:refnum<file>, error out=w1365:errorcluster)
            n905 = Close File(refnum=w1366, error in=w1365) -> ()  [unwired: 2 out]
          }
        }
      }
      event "模型": Value Change {
        n906 = event-data() -> ()  [unwired: 1 in, 6 out]
        n907 = global read "COD内部交互全局.vi" "配置文件ini"() -> (w1376:string)
        n908 = call <vilib>:"Application Directory.vi"() -> ("Application Directory"=w1385:path)
        n909 = Build Path(base path=w1385, name or relative path=w1376) -> (appended path=w1384:path)
        n910 = call <vilib>:"Open Config Data.vi"("configuration file path"=w1384) -> ("error out"=w1382:errorcluster, "refnum"=w1383:T3)  [unwired: 8 in, 1 out]
        n911 = local read "模型"() -> (w1377:enum32{"线性", "多项式"})
        n912 = call-poly <vilib>:"Write Key.vi"("section"="CODMn模型选择" ("key"), "error in (no error)"=w1382, "value"=w1377, "key"="线性和多项式", "refnum"=w1383) -> ("error out"=w1378:errorcluster, "refnum out"=w1379:T3)  [unwired: 4 in, 1 out]
        n913 = call <vilib>:"Close Config Data.vi"("error in (no error)"=w1378, "refnum"=w1379) -> ()  [unwired: 8 in, 2 out]
      }
      event "浓度1", "浓度2", "浓度3", "泵滴定数1", "泵滴定数2", "泵滴定数3", "启用1", "启用2", "启用3", "浓度4", "浓度5", "泵滴定数4", "泵滴定数5", "启用4", "启用5": Value Change {
        n914 = event-data() -> ()  [unwired: 1 in, 6 out]
        n915 = global read "COD内部交互全局.vi" "配置文件ini"() -> (w1386:string)
        n916 = local read "选用水样"() -> (w1402:enum16{"葡萄糖", "草酸钠"})
        n917 = local read "量程选择"() -> (w1401:enum16{"低量程", "高量程", "0-2量程"})
        n918 = call <vilib>:"Application Directory.vi"() -> ("Application Directory"=w1460:path)
        n919 = case shown="\"葡萄糖\", 默认" w1402 {
          tunnel: ["葡萄糖标线" ("section") "草酸钠标线" ("section")] -> w1408
          frame "葡萄糖", Default {
          }
          frame "草酸钠" {
          }
        }
        n920 = Build Path(base path=w1460, name or relative path=w1386) -> (appended path=w1459:path)
        n921 = case shown="\"0-2量程\"" w1401 {
          tunnel: ["低量程" "高量程" "0-2量程"] -> w1399
          frame "低量程", Default {
          }
          frame "高量程" {
          }
          frame "0-2量程" {
          }
        }
        n922 = Concatenate Strings(w1408, w1399) -> (w1400:string)
        n923 = call <vilib>:"Open Config Data.vi"("configuration file path"=w1459) -> ("error out"=w1457:errorcluster, "refnum"=w1458:T3)  [unwired: 8 in, 1 out]
        n924 = local read "浓度1"() -> (w1455:dbl)
        n925 = call-poly <vilib>:"Write Key.vi"("section"=w1400, "error in (no error)"=w1457, "value"=w1455, "key"="浓度1", "refnum"=w1458) -> ("error out"=w1454:errorcluster, "refnum out"=w1453:T3)  [unwired: 4 in, 1 out]
        n926 = local read "浓度2"() -> (w1439:dbl)
        n927 = call-poly <vilib>:"Write Key.vi"("section"=w1400, "error in (no error)"=w1454, "value"=w1439, "key"="浓度2", "refnum"=w1453) -> ("error out"=w1452:errorcluster, "refnum out"=w1451:T3)  [unwired: 4 in, 1 out]
        n928 = local read "浓度3"() -> (w1435:dbl)
        n929 = local read "泵滴定数1"() -> (w1433:dbl)
        n930 = call-poly <vilib>:"Write Key.vi"("section"=w1400, "error in (no error)"=w1452, "value"=w1435, "key"="浓度3", "refnum"=w1451) -> ("error out"=w1450:errorcluster, "refnum out"=w1449:T3)  [unwired: 4 in, 1 out]
        n931 = local read "泵滴定数2"() -> (w1431:dbl)
        n932 = call-poly <vilib>:"Write Key.vi"("section"=w1400, "error in (no error)"=w1450, "value"=w1433, "key"="泵滴定数1", "refnum"=w1449) -> ("error out"=w1448:errorcluster, "refnum out"=w1447:T3)  [unwired: 4 in, 1 out]
        n933 = local read "泵滴定数3"() -> (w1429:dbl)
        n934 = call-poly <vilib>:"Write Key.vi"("section"=w1400, "error in (no error)"=w1448, "value"=w1431, "key"="泵滴定数2", "refnum"=w1447) -> ("error out"=w1446:errorcluster, "refnum out"=w1445:T3)  [unwired: 4 in, 1 out]
        n935 = call-poly <vilib>:"Write Key.vi"("section"=w1400, "error in (no error)"=w1446, "value"=w1429, "key"="泵滴定数3", "refnum"=w1445) -> ("error out"=w1444:errorcluster, "refnum out"=w1443:T3)  [unwired: 4 in, 1 out]
        n936 = local read "浓度4"() -> (w1398:dbl)
        n937 = call-poly <vilib>:"Write Key.vi"("section"=w1400, "error in (no error)"=w1444, "value"=w1398, "key"="浓度4", "refnum"=w1443) -> ("error out"=w1437:errorcluster, "refnum out"=w1438:T3)  [unwired: 4 in, 1 out]
        n938 = local read "浓度5"() -> (w1397:dbl)
        n939 = local read "泵滴定数4"() -> (w1394:dbl)
        n940 = call-poly <vilib>:"Write Key.vi"("section"=w1400, "error in (no error)"=w1437, "value"=w1397, "key"="浓度5", "refnum"=w1438) -> ("error out"=w1395:errorcluster, "refnum out"=w1396:T3)  [unwired: 4 in, 1 out]
        n941 = local read "泵滴定数5"() -> (w1393:dbl)
        n942 = call-poly <vilib>:"Write Key.vi"("section"=w1400, "error in (no error)"=w1395, "value"=w1394, "key"="泵滴定数4", "refnum"=w1396) -> ("error out"=w1442:errorcluster, "refnum out"=w1441:T3)  [unwired: 4 in, 1 out]
        n943 = call-poly <vilib>:"Write Key.vi"("section"=w1400, "error in (no error)"=w1442, "value"=w1393, "key"="泵滴定数5", "refnum"=w1441) -> ("error out"=w1391:errorcluster, "refnum out"=w1392:T3)  [unwired: 4 in, 1 out]
        n944 = local read "启用1"() -> (w1417:bool)
        n945 = call-poly <vilib>:"Write Key.vi"("section"=w1400, "error in (no error)"=w1391, "value"=w1417, "key"="启用1", "refnum"=w1392) -> ("error out"=w1413:errorcluster, "refnum out"=w1416:T3)  [unwired: 4 in, 1 out]
        n946 = local read "启用2"() -> (w1414:bool)
        n947 = call-poly <vilib>:"Write Key.vi"("section"=w1400, "error in (no error)"=w1413, "value"=w1414, "key"="启用2", "refnum"=w1416) -> ("error out"=w1424:errorcluster, "refnum out"=w1423:T3)  [unwired: 4 in, 1 out]
        n948 = local read "启用3"() -> (w1412:bool)
        n949 = call-poly <vilib>:"Write Key.vi"("section"=w1400, "error in (no error)"=w1424, "value"=w1412, "key"="启用3", "refnum"=w1423) -> ("error out"=w1422:errorcluster, "refnum out"=w1421:T3)  [unwired: 4 in, 1 out]
        n950 = local read "启用4"() -> (w1387:bool)
        n951 = call-poly <vilib>:"Write Key.vi"("section"=w1400, "error in (no error)"=w1422, "value"=w1387, "key"="启用4", "refnum"=w1421) -> ("error out"=w1420:errorcluster, "refnum out"=w1419:T3)  [unwired: 4 in, 1 out]
        n952 = local read "启用5"() -> (w1388:bool)
        n953 = local read "选用水样"() -> (w1407:enum16{"葡萄糖", "草酸钠"})
        n954 = call-poly <vilib>:"Write Key.vi"("section"=w1400, "error in (no error)"=w1420, "value"=w1388, "key"="启用5", "refnum"=w1419) -> ("error out"=w1389:errorcluster, "refnum out"=w1390:T3)  [unwired: 4 in, 1 out]
        n955 = call-poly <vilib>:"Write Key.vi"("section"="标线选择", "error in (no error)"=w1389, "value"=w1407, "key"="选用水样", "refnum"=w1390) -> ("error out"=w1404:errorcluster, "refnum out"=w1405:T3)  [unwired: 4 in, 1 out]
        n956 = call <vilib>:"Close Config Data.vi"("error in (no error)"=w1404, "refnum"=w1405) -> ()  [unwired: 8 in, 2 out]
      }
      event "读取": Value Change {
        (unwired) u16 94 ("number of holding registers")
        (unwired) u16 4616 ("starting address")
        n957 = event-data() -> ()  [unwired: 1 in, 6 out]
        n958 = Bundle By Name(cluster=cluster{"命令":string} {"命令"=""} ("元素"), "命令"="CODMn读取公式" ("名称（未命名）")) -> (w1466:cluster{"命令":string})
        n959 = Enqueue Element(queue=w1470, element=w1466, error in (no error)=w1469) -> ()  [unwired: 1 in, 3 out]
      }
      event "写入": Mouse Down {
        n960 = event-data() -> ()  [unwired: 1 in, 8 out]
        n961 = Two Button Dialog(message="是否将上方方程系数K、B、X^2的值写入，写入会覆盖原有公式！" ("消息")) -> (T button?=w1471:bool)  [unwired: 2 in]
        n962 = case shown="真" w1471 {
          frame False {
          }
          frame True {
            n963 = local read "模型"() -> (w1482:enum32{"线性", "多项式"})
            n964 = case shown="\"多项式\"" w1482 {
              tunnel: [w1511 w1555] -> w1480
              tunnel: [w1510 w1554] -> w1479
              frame "线性", Default {
                (unwired) "线性" ("table输入")
                n965 = local read "测量模式(公式)"() -> (w1512:u16)
                n966 = case shown="1" w1512 {
                  tunnel: [u16 4626 ("starting address") w1519 w1524 w1529 w1534 w1539 w1544 w1549] -> w1511
                  frame 0, Default {
                  }
                  frame 1 {
                    n967 = local read "量程选择"() -> (w1518:enum16{"低量程", "高量程", "0-2量程"})
                    n968 = case shown="\"低量程\", 默认" w1518 {
                      tunnel: [u16 4626 ("starting address") u16 4632 ("starting address") u16 4638 ("starting address")] -> w1519
                      frame "低量程", Default {
                      }
                      frame "高量程" {
                      }
                      frame "0-2量程" {
                      }
                    }
                  }
                  frame 2 {
                    n969 = local read "量程选择"() -> (w1523:enum16{"低量程", "高量程", "0-2量程"})
                    n970 = case shown="\"低量程\", 默认" w1523 {
                      tunnel: [u16 4638 ("starting address") u16 4644 ("starting address") u16 4638 ("starting address")] -> w1524
                      frame "低量程", Default {
                      }
                      frame "高量程" {
                      }
                      frame "0-2量程" {
                      }
                    }
                  }
                  frame 3 {
                    n971 = local read "量程选择"() -> (w1528:enum16{"低量程", "高量程", "0-2量程"})
                    n972 = case shown="\"低量程\", 默认" w1528 {
                      tunnel: [u16 4650 ("starting address") u16 4656 ("starting address") u16 4638 ("starting address")] -> w1529
                      frame "低量程", Default {
                      }
                      frame "高量程" {
                      }
                      frame "0-2量程" {
                      }
                    }
                  }
                  frame 4 {
                    n973 = local read "量程选择"() -> (w1533:enum16{"低量程", "高量程", "0-2量程"})
                    n974 = case shown="\"低量程\", 默认" w1533 {
                      tunnel: [u16 4662 ("starting address") u16 4668 ("starting address") u16 4638 ("starting address")] -> w1534
                      frame "低量程", Default {
                      }
                      frame "高量程" {
                      }
                      frame "0-2量程" {
                      }
                    }
                  }
                  frame 5 {
                    n975 = local read "量程选择"() -> (w1538:enum16{"低量程", "高量程", "0-2量程"})
                    n976 = case shown="\"低量程\", 默认" w1538 {
                      tunnel: [u16 4674 ("starting address") u16 4680 ("starting address") u16 4638 ("starting address")] -> w1539
                      frame "低量程", Default {
                      }
                      frame "高量程" {
                      }
                      frame "0-2量程" {
                      }
                    }
                  }
                  frame 6 {
                    n977 = local read "量程选择"() -> (w1543:enum16{"低量程", "高量程", "0-2量程"})
                    n978 = case shown="\"低量程\", 默认" w1543 {
                      tunnel: [u16 4686 ("starting address") u16 4692 ("starting address") u16 4638 ("starting address")] -> w1544
                      frame "低量程", Default {
                      }
                      frame "高量程" {
                      }
                      frame "0-2量程" {
                      }
                    }
                  }
                  frame 7 {
                    n979 = local read "量程选择"() -> (w1548:enum16{"低量程", "高量程", "0-2量程"})
                    n980 = case shown="\"低量程\", 默认" w1548 {
                      tunnel: [u16 4698 ("starting address") u16 4704 ("starting address") u16 4638 ("starting address")] -> w1549
                      frame "低量程", Default {
                      }
                      frame "高量程" {
                      }
                      frame "0-2量程" {
                      }
                    }
                  }
                }
                n981 = local read "K"() -> (w1516:dbl)
                n982 = local read "b"() -> (w1515:dbl)
                n983 = Build Array(w1516, w1515, 0.0 ("元素")) -> (w1514:dbl[])
                n984 = call "浮点转CDAB整形cod.vi"("浮点数"=w1514) -> ("CDAB整形输出"=w1510:u16[])  [unwired: 10 in]
              }
              frame "多项式" {
                (unwired) "多项式" ("table输入")
                # "b,k,c"
                n985 = local read "多项式系数"() -> (w1560:dbl[])
                n986 = local read "测量模式(公式)"() -> (w1556:u16)
                n987 = Index Array(array=w1560) -> (element #1=w1558:dbl, element #2=w1553:dbl, element #3=w1557:dbl)  [unwired: 3 in]
                n988 = case shown="1" w1556 {
                  tunnel: [u16 4626 ("starting address") w1563 w1568 w1573 w1578 w1583 w1588 w1593] -> w1555
                  frame 0, Default {
                  }
                  frame 1 {
                    n989 = local read "量程选择"() -> (w1562:enum16{"低量程", "高量程", "0-2量程"})
                    n990 = case shown="\"低量程\", 默认" w1562 {
                      tunnel: [u16 4626 ("starting address") u16 4632 ("starting address") u16 4638 ("starting address")] -> w1563
                      frame "低量程", Default {
                      }
                      frame "高量程" {
                      }
                      frame "0-2量程" {
                      }
                    }
                  }
                  frame 2 {
                    n991 = local read "量程选择"() -> (w1567:enum16{"低量程", "高量程", "0-2量程"})
                    n992 = case shown="\"低量程\", 默认" w1567 {
                      tunnel: [u16 4638 ("starting address") u16 4644 ("starting address") u16 4638 ("starting address")] -> w1568
                      frame "低量程", Default {
                      }
                      frame "高量程" {
                      }
                      frame "0-2量程" {
                      }
                    }
                  }
                  frame 3 {
                    n993 = local read "量程选择"() -> (w1572:enum16{"低量程", "高量程", "0-2量程"})
                    n994 = case shown="\"低量程\", 默认" w1572 {
                      tunnel: [u16 4650 ("starting address") u16 4656 ("starting address") u16 4638 ("starting address")] -> w1573
                      frame "低量程", Default {
                      }
                      frame "高量程" {
                      }
                      frame "0-2量程" {
                      }
                    }
                  }
                  frame 4 {
                    n995 = local read "量程选择"() -> (w1577:enum16{"低量程", "高量程", "0-2量程"})
                    n996 = case shown="\"低量程\", 默认" w1577 {
                      tunnel: [u16 4662 ("starting address") u16 4668 ("starting address") u16 4638 ("starting address")] -> w1578
                      frame "低量程", Default {
                      }
                      frame "高量程" {
                      }
                      frame "0-2量程" {
                      }
                    }
                  }
                  frame 5 {
                    n997 = local read "量程选择"() -> (w1582:enum16{"低量程", "高量程", "0-2量程"})
                    n998 = case shown="\"低量程\", 默认" w1582 {
                      tunnel: [u16 4674 ("starting address") u16 4680 ("starting address") u16 4638 ("starting address")] -> w1583
                      frame "低量程", Default {
                      }
                      frame "高量程" {
                      }
                      frame "0-2量程" {
                      }
                    }
                  }
                  frame 6 {
                    n999 = local read "量程选择"() -> (w1587:enum16{"低量程", "高量程", "0-2量程"})
                    n1000 = case shown="\"低量程\", 默认" w1587 {
                      tunnel: [u16 4686 ("starting address") u16 4692 ("starting address") u16 4638 ("starting address")] -> w1588
                      frame "低量程", Default {
                      }
                      frame "高量程" {
                      }
                      frame "0-2量程" {
                      }
                    }
                  }
                  frame 7 {
                    n1001 = local read "量程选择"() -> (w1592:enum16{"低量程", "高量程", "0-2量程"})
                    n1002 = case shown="\"低量程\", 默认" w1592 {
                      tunnel: [u16 4698 ("starting address") u16 4704 ("starting address") u16 4638 ("starting address")] -> w1593
                      frame "低量程", Default {
                      }
                      frame "高量程" {
                      }
                      frame "0-2量程" {
                      }
                    }
                  }
                }
                n1003 = Build Array(w1553, w1558, w1557) -> (w1559:dbl[])
                n1004 = call "浮点转CDAB整形cod.vi"("浮点数"=w1559) -> ("CDAB整形输出"=w1554:u16[])  [unwired: 10 in]
              }
            }
            n1005 = local read "多项式系数"() -> (w1476:dbl[])
            n1006 = call "CODMnMB_api.vi"("STEP"=enum16{"open", "read", "write", "close"}."write", "values"=w1479, "starting address"=w1480) -> ("error out"=w1478:errorcluster)  [unwired: 6 in, 2 out]
            n1007 = Index Array(array=w1476) -> (element #1=w1475:dbl, element #2=w1474:dbl, element #3=w1473:dbl)  [unwired: 3 in]
            n1008 = case shown="无错误" w1478 {
              tunnel: ["写入成功！" "写入失败！"] -> w1477
              tunnel: w1475 -> [w1488 _]
              tunnel: w1474 -> [w1487 _]
              tunnel: w1473 -> [w1486 _]
              frame No Error {
                n1009 = Number To Fractional String(number=w1488) -> (F-format string=w1484:string)  [unwired: 3 in]
                n1010 = Number To Fractional String(number=w1487) -> (F-format string=w1485:string)  [unwired: 3 in]
                n1011 = Number To Fractional String(number=w1486) -> (F-format string=w1483:string)  [unwired: 3 in]
                n1012 = property on="模型" class="Enum (严格)"() -> ("RingText.Text"=w1498:string)  [unwired: 2 in, 2 out]
                n1013 = property on="测量模式(公式)" class="Ring (严格)"() -> ("RingText.Text"=w1497:string)  [unwired: 2 in, 2 out]
                n1014 = property on="量程选择" class="Enum (严格)"() -> ("RingText.Text"=w1496:string)  [unwired: 2 in, 2 out]
                n1015 = Concatenate Strings("变更后:" ("table输入"), "K:" ("字符串"), w1485, "B:" ("字符串"), w1484, "X^2:" ("字符串"), w1483) -> (w1489:string)
                n1016 = Concatenate Strings(w1498, w1497, w1496, "公式改变" ("日志信息")) -> (w1490:string)
                n1017 = Get Date/Time In Seconds() -> (seconds since 1Jan1904=w1502:timestamp)
                n1018 = Bundle(cluster=T12 {"时间标识"=timestamp(0 s since 1904-01-01), "参数"="", "日志信息"="", "流程参数"=""} ("data in"), "时间标识"=w1502, "参数"="CODMn" ("table输入"), "日志信息"=w1490, "流程参数"=w1489) -> (w1500:T12)
                n1019 = call "流程日志字段定义.vi"("table输入"="操作日志", "data in"=w1500) -> ("table输出"=w1505:string, "columns"=w1506:string[], "data out"=w1507:T14)  [unwired: 7 in]
                n1020 = call "插入数据.vi"("data"=w1507, "columns"=w1506, "database"="database3.mdb", "table"=w1505) -> ()  [unwired: 7 in, 1 out]
              }
              frame Error {
              }
            }
            n1021 = One Button Dialog(message=w1477) -> ()  [unwired: 1 in, 1 out]
          }
        }
      }
      event "一键写入": Value Change {
        n1022 = event-data() -> ()  [unwired: 1 in, 6 out]
        n1023 = Two Button Dialog(message="确认是否写入公式，写入会覆盖原有公式！" ("消息")) -> (T button?=w1597:bool)  [unwired: 2 in]
        n1024 = case shown="真" w1597 {
          frame False {
          }
          frame True {
            n1025 = local read "模型"() -> (w1601:enum32{"线性", "多项式"})
            n1026 = case shown="\"多项式\"" w1601 {
              tunnel: [w1604 w1655] -> w1599
              frame "线性", Default {
                n1027 = property on="测量模式(公式)" class="Ring (严格)"() -> ("NumItems"=w1605:u32)  [unwired: 2 in, 2 out]
                n1028 = for {
                  N: w1605 -> [_]
                  tunnel: [w1606] -> w1604
                  i -> [w1611]
                  n1029 = Increment(x=w1611) -> (x+1=w1610:i32)
                  n1030 = local read "K"() -> (w1615:dbl)
                  n1031 = local read "b"() -> (w1616:dbl)
                  n1032 = case shown="1" w1610 {
                    tunnel: [u16 4626 ("starting address") w1621 w1626 w1631 w1636 w1641 w1646 w1651] -> w1608
                    frame 0, Default {
                    }
                    frame 1 {
                      n1033 = local read "量程选择"() -> (w1620:enum16{"低量程", "高量程", "0-2量程"})
                      n1034 = case shown="\"低量程\", 默认" w1620 {
                        tunnel: [u16 4626 ("starting address") u16 4632 ("starting address") u16 4638 ("starting address")] -> w1621
                        frame "低量程", Default {
                        }
                        frame "高量程" {
                        }
                        frame "0-2量程" {
                        }
                      }
                    }
                    frame 2 {
                      n1035 = local read "量程选择"() -> (w1625:enum16{"低量程", "高量程", "0-2量程"})
                      n1036 = case shown="\"低量程\", 默认" w1625 {
                        tunnel: [u16 4638 ("starting address") u16 4644 ("starting address") u16 4638 ("starting address")] -> w1626
                        frame "低量程", Default {
                        }
                        frame "高量程" {
                        }
                        frame "0-2量程" {
                        }
                      }
                    }
                    frame 3 {
                      n1037 = local read "量程选择"() -> (w1630:enum16{"低量程", "高量程", "0-2量程"})
                      n1038 = case shown="\"低量程\", 默认" w1630 {
                        tunnel: [u16 4650 ("starting address") u16 4656 ("starting address") u16 4638 ("starting address")] -> w1631
                        frame "低量程", Default {
                        }
                        frame "高量程" {
                        }
                        frame "0-2量程" {
                        }
                      }
                    }
                    frame 4 {
                      n1039 = local read "量程选择"() -> (w1635:enum16{"低量程", "高量程", "0-2量程"})
                      n1040 = case shown="\"高量程\"" w1635 {
                        tunnel: [u16 4662 ("starting address") u16 4668 ("starting address") u16 4638 ("starting address")] -> w1636
                        frame "低量程", Default {
                        }
                        frame "高量程" {
                        }
                        frame "0-2量程" {
                        }
                      }
                    }
                    frame 5 {
                      n1041 = local read "量程选择"() -> (w1640:enum16{"低量程", "高量程", "0-2量程"})
                      n1042 = case shown="\"低量程\", 默认" w1640 {
                        tunnel: [u16 4674 ("starting address") u16 4680 ("starting address") u16 4638 ("starting address")] -> w1641
                        frame "低量程", Default {
                        }
                        frame "高量程" {
                        }
                        frame "0-2量程" {
                        }
                      }
                    }
                    frame 6 {
                      n1043 = local read "量程选择"() -> (w1645:enum16{"低量程", "高量程", "0-2量程"})
                      n1044 = case shown="\"低量程\", 默认" w1645 {
                        tunnel: [u16 4686 ("starting address") u16 4692 ("starting address") u16 4638 ("starting address")] -> w1646
                        frame "低量程", Default {
                        }
                        frame "高量程" {
                        }
                        frame "0-2量程" {
                        }
                      }
                    }
                    frame 7 {
                      n1045 = local read "量程选择"() -> (w1650:enum16{"低量程", "高量程", "0-2量程"})
                      n1046 = case shown="\"低量程\", 默认" w1650 {
                        tunnel: [u16 4698 ("starting address") u16 4704 ("starting address") u16 4638 ("starting address")] -> w1651
                        frame "低量程", Default {
                        }
                        frame "高量程" {
                        }
                        frame "0-2量程" {
                        }
                      }
                    }
                  }
                  n1047 = Build Array(w1615, w1616, 0.0 ("元素")) -> (w1617:dbl[])
                  n1048 = call "浮点转CDAB整形cod.vi"("浮点数"=w1617) -> ("CDAB整形输出"=w1614:u16[])  [unwired: 10 in]
                  n1049 = Insert Into Array(array=u16[] [], index=0 ("索引"), new element=w1614) -> (w1607:u16[])
                  n1050 = call "CODMnMB_api.vi"("STEP"=enum16{"open", "read", "write", "close"}."write", "values"=w1607, "starting address"=w1608) -> ("error out"=w1606:errorcluster)  [unwired: 6 in, 2 out]
                }
              }
              frame "多项式" {
                # "b,k,c"
                n1051 = property on="测量模式(公式)" class="Ring (严格)"() -> ("NumItems"=w1656:u32)  [unwired: 2 in, 2 out]
                n1052 = for {
                  N: w1656 -> [_]
                  tunnel: [w1657] -> w1655
                  i -> [w1662]
                  n1053 = Increment(x=w1662) -> (x+1=w1661:i32)
                  n1054 = local read "多项式系数"() -> (w1666:dbl[])
                  n1055 = case shown="2" w1661 {
                    tunnel: [u16 4626 ("starting address") w1673 w1678 w1683 w1688 w1693 w1698 w1703] -> w1658
                    frame 0, Default {
                    }
                    frame 1 {
                      n1056 = local read "量程选择"() -> (w1672:enum16{"低量程", "高量程", "0-2量程"})
                      n1057 = case shown="\"低量程\", 默认" w1672 {
                        tunnel: [u16 4626 ("starting address") u16 4632 ("starting address") u16 4638 ("starting address")] -> w1673
                        frame "低量程", Default {
                        }
                        frame "高量程" {
                        }
                        frame "0-2量程" {
                        }
                      }
                    }
                    frame 2 {
                      n1058 = local read "量程选择"() -> (w1677:enum16{"低量程", "高量程", "0-2量程"})
                      n1059 = case shown="\"低量程\", 默认" w1677 {
                        tunnel: [u16 4638 ("starting address") u16 4644 ("starting address") u16 4638 ("starting address")] -> w1678
                        frame "低量程", Default {
                        }
                        frame "高量程" {
                        }
                        frame "0-2量程" {
                        }
                      }
                    }
                    frame 3 {
                      n1060 = local read "量程选择"() -> (w1682:enum16{"低量程", "高量程", "0-2量程"})
                      n1061 = case shown="\"低量程\", 默认" w1682 {
                        tunnel: [u16 4650 ("starting address") u16 4656 ("starting address") u16 4638 ("starting address")] -> w1683
                        frame "低量程", Default {
                        }
                        frame "高量程" {
                        }
                        frame "0-2量程" {
                        }
                      }
                    }
                    frame 4 {
                      n1062 = local read "量程选择"() -> (w1687:enum16{"低量程", "高量程", "0-2量程"})
                      n1063 = case shown="\"低量程\", 默认" w1687 {
                        tunnel: [u16 4662 ("starting address") u16 4668 ("starting address") u16 4638 ("starting address")] -> w1688
                        frame "低量程", Default {
                        }
                        frame "高量程" {
                        }
                        frame "0-2量程" {
                        }
                      }
                    }
                    frame 5 {
                      n1064 = local read "量程选择"() -> (w1692:enum16{"低量程", "高量程", "0-2量程"})
                      n1065 = case shown="\"低量程\", 默认" w1692 {
                        tunnel: [u16 4674 ("starting address") u16 4680 ("starting address") u16 4638 ("starting address")] -> w1693
                        frame "低量程", Default {
                        }
                        frame "高量程" {
                        }
                        frame "0-2量程" {
                        }
                      }
                    }
                    frame 6 {
                      n1066 = local read "量程选择"() -> (w1697:enum16{"低量程", "高量程", "0-2量程"})
                      n1067 = case shown="\"低量程\", 默认" w1697 {
                        tunnel: [u16 4686 ("starting address") u16 4692 ("starting address") u16 4638 ("starting address")] -> w1698
                        frame "低量程", Default {
                        }
                        frame "高量程" {
                        }
                        frame "0-2量程" {
                        }
                      }
                    }
                    frame 7 {
                      n1068 = local read "量程选择"() -> (w1702:enum16{"低量程", "高量程", "0-2量程"})
                      n1069 = case shown="\"低量程\", 默认" w1702 {
                        tunnel: [u16 4698 ("starting address") u16 4704 ("starting address") u16 4638 ("starting address")] -> w1703
                        frame "低量程", Default {
                        }
                        frame "高量程" {
                        }
                        frame "0-2量程" {
                        }
                      }
                    }
                  }
                  n1070 = Index Array(array=w1666) -> (element #1=w1669:dbl, element #2=w1668:dbl, element #3=w1670:dbl)  [unwired: 3 in]
                  n1071 = Build Array(w1668, w1669, w1670) -> (w1667:dbl[])
                  n1072 = call "浮点转CDAB整形cod.vi"("浮点数"=w1667) -> ("CDAB整形输出"=w1665:u16[])  [unwired: 10 in]
                  n1073 = Insert Into Array(array=u16[] [], index=0 ("索引"), new element=w1665) -> (w1659:u16[])
                  n1074 = call "CODMnMB_api.vi"("STEP"=enum16{"open", "read", "write", "close"}."write", "values"=w1659, "starting address"=w1658) -> ("error out"=w1657:errorcluster)  [unwired: 6 in, 2 out]
                }
              }
            }
            n1075 = case shown="无错误" w1599 {
              tunnel: ["写入成功！" "写入失败！"] -> w1600
              frame No Error {
              }
              frame Error {
              }
            }
            n1076 = One Button Dialog(message=w1600) -> ()  [unwired: 1 in, 1 out]
          }
        }
      }
      event "滴定曲线": Value Change {
        n1077 = event-data() -> ()  [unwired: 1 in, 6 out]
        n1078 = property on="窗格" class="Pane"("Origin"=T2 {"Horizontal"=0, "Vertical"=3200} ("原点")) -> ()  [unwired: 2 in, 2 out]
      }
      event "历史波形": Value Change {
        n1079 = event-data() -> ()  [unwired: 1 in, 6 out]
        n1080 = call-poly <vilib>:"Read Waveforms from File.vi"() -> ("error out"=w1708:errorcluster, "first waveform in record"=w1709:waveform(dbl))  [unwired: 6 in, 2 out]
        n1081 = case shown="无错误" w1708 {
          tunnel: w1709 -> [w1712 _]
          frame No Error {
            n1082 = Unbundle By Name(w1712) -> ("t0"=→"波形时间":timestamp, "Y"=w1711:dbl[])  [unwired: 2 out]
            n1083 = local write "ORP滴定曲线"(w1711) -> ()
            n1084 = local write "滴定数-ORP值"(w1711) -> ()
          }
          frame Error {
            n1085 = One Button Dialog(message="打开失败" ("消息")) -> ()  [unwired: 1 in, 1 out]
          }
        }
      }
      event "释放串口": Value Change {
        n1086 = event-data() -> ()  [unwired: 1 in, 6 out]
        n1087 = Two Button Dialog(message="确认是否释放串口，释放串口将导致通信失败！" ("消息")) -> (T button?=w1714:bool)  [unwired: 2 in]
        n1088 = case shown="真" w1714 {
          tunnel: w1717 -> [_ w1719]
          tunnel: w1716 -> [_ w1718]
          frame False {
          }
          frame True {
            n1089 = Bundle By Name(cluster=cluster{"命令":string} {"命令"=""} ("元素"), "命令"="停用模块" ("名称（未命名）")) -> (w1720:cluster{"命令":string})
            n1090 = Enqueue Element(queue=w1719, element=w1720, error in (no error)=w1718) -> ()  [unwired: 1 in, 3 out]
          }
        }
      }
      event "打开串口": Value Change {
        n1091 = event-data() -> ()  [unwired: 1 in, 6 out]
        n1092 = flat-sequence {
          tunnel: w1724 -> [w1732]
          tunnel: w1723 -> [w1731]
          frame #0 {
            n1093 = global read "CODMn断电保存全局变量.vi" "VISA resource name"() -> (w1735:refnum<visa-resource-name>)
            n1094 = global read "CODMn断电保存全局变量.vi" "MB通信方式选择"() -> (w1728:enum16{"串口", "TCP"})
            n1095 = global read "CODMn断电保存全局变量.vi" "PORT"() -> (w1726:string)
            n1096 = global read "CODMn断电保存全局变量.vi" "IP"() -> (w1727:string)
            n1097 = call "串口配置.vi"("PORT"=w1726, "IP"=w1727, "MB通信方式选择"=w1728, "请选择串口:"=w1735) -> ("PORT 2"=w1729:string, "IP 2"=w1730:string, "确认 2"=w1733:bool, "VISA资源名称 2"=w1734:refnum<visa-resource-name>, "MB通信方式选择 2"=w1725:enum16{"串口", "TCP"})  [unwired: 3 in]
            n1098 = case shown="真" w1733 {
              tunnel: w1734 -> [_ w1744]
              tunnel: w1732 -> [_ w1740]
              tunnel: w1731 -> [_ w1739]
              tunnel: w1730 -> [_ w1738]
              tunnel: w1729 -> [_ w1737]
              tunnel: w1725 -> [_ w1736]
              frame False {
              }
              frame True {
                n1099 = global write "CODMn断电保存全局变量.vi" "IP"(w1738) -> ()
                n1100 = global write "CODMn断电保存全局变量.vi" "PORT"(w1737) -> ()
                n1101 = global write "CODMn断电保存全局变量.vi" "VISA resource name"(w1744) -> ()
                n1102 = global write "CODMn断电保存全局变量.vi" "MB通信方式选择"(w1736) -> ()
                n1103 = Bundle By Name(cluster=cluster{"命令":string} {"命令"=""} ("元素"), "命令"="启用模块" ("名称（未命名）")) -> (w1741:cluster{"命令":string})
                n1104 = Enqueue Element(queue=w1740, element=w1741, error in (no error)=w1739) -> ()  [unwired: 1 in, 3 out]
              }
            }
          }
          frame #1 {
            n1105 = global read "COD内部交互全局.vi" "配置文件ini"() -> (w1758:string)
            n1106 = call <vilib>:"Application Directory.vi"() -> ("Application Directory"=w1745:path)
            n1107 = Build Path(base path=w1745, name or relative path=w1758) -> (appended path=w1746:path)
            n1108 = call <vilib>:"Open Config Data.vi"("configuration file path"=w1746) -> ("error out"=w1750:errorcluster, "refnum"=w1747:T3)  [unwired: 8 in, 1 out]
            n1109 = vi-ref "斯坦道CODMn.lvlib:CODMn断电保存全局变量.vi"() -> (w1748:refnum<vi>)
            n1110 = call <userlib>:"Write Panel to INI__ogtk.vi"("error in (no error)"=w1750, "VI ref"=w1748, "refnum"=w1747) -> ("error out"=w1751:errorcluster, "refnum out"=w1749:T3)  [unwired: 7 in]
            n1111 = call <vilib>:"Close Config Data.vi"("error in (no error)"=w1751, "refnum"=w1749) -> ("error out"=w1756:errorcluster, "file path"=w1757:path)  [unwired: 8 in]
            n1112 = Open/Create/Replace File(file path (use dialog)=w1757, error in=w1756) -> (refnum out=w1753:refnum<file>, error out=w1752:errorcluster)  [unwired: 4 in, 1 out]
            n1113 = Flush File(refnum=w1753, error in=w1752) -> (refnum out=w1754:refnum<file>, error out=w1755:errorcluster)
            n1114 = Close File(refnum=w1754, error in=w1755) -> ()  [unwired: 2 out]
          }
        }
      }
      event Timeout {
        n1115 = event-data() -> ()  [unwired: 1 in, 3 out]
      }
    }
  }
  n1116 = property class="VI"(reference=w38, error in=w37) -> ("Name"=w40:string)  [unwired: 2 out]
  n1117 = Open VI Reference(type specifier VI Refnum (for type only)=refnum<vi> refnum, vi path=w40, options=128 ("选项")) -> (vi reference=w42:refnum<vi>, error out=w44:errorcluster)  [unwired: 3 in]
  n1118 = call-by-ref "?"(reference=w42, error in=w44) -> (reference out=w46:refnum<vi>, error out=w45:errorcluster)  [unwired: 12 in]
  n1119 = Close Reference(reference=w46, error in (no error)=w45) -> ()  [unwired: 1 out]
